vi "Auto.vi"() -> ()   [LabVIEW 2020]
uses:
  Global_Variable/A180648.vi
  Global_Variable/Global.vi
  Global_Variable/excursion.vi
  <userlib>/_MGI/1D Array/MGI Running Average/MGI Running Average(DBL).vi
  <userlib>/_MGI/1D Array/MGI Running Average/MGI Running Average(SGL).vi
  <userlib>/_MGI/1D Array/MGI Average/MGI Average (DBL[][]).vi
  Libraries/S7/S7.lvlib
  <vilib>/ptbypt/NI_PtbyPt.lvlib
panel:
  out "可信度检测":cluster{dbl[], dbl[]}[](graph)
  out "传感器特性":cluster{dbl[], dbl[]}[](graph)
  in  "error in (no error)":errorcluster caption="错误输入（无错误）"
  out "初始角度":dbl
  out "T1-T2_135°":dbl
  out "T1-T2_225°":dbl
  out "T1-T2_315°":dbl
  out "T1-T2_360°":dbl
  out "T1-T2_270°":dbl
  out "T1-T2_180°":dbl
  out "T1-T2_45°":dbl
  out "T1-T2_90°":dbl
  out "初始化 3":bool[](array[boolean])
  out "动优化态前":cluster{dbl[], dbl[]}[](graph)
  in  "initialize 2":bool caption="初始化"
  in  "initialize":bool caption="初始化"
  out "vRES_cCW":cluster{dbl[], dbl[]}
  out "VRES_cW":cluster{dbl[], dbl[]}
  out "初始化 2":bool[](array[boolean])
  in  "选项卡控件":enum32{"工位一程序复检", "工位一动态复检"}(tab)
  in  "请启动":bool
  out "Vres_45°":dbl format="%#.6f"
  out "Vres_135°":dbl format="%#.6f"
  out "Vres_225°":dbl format="%#.6f"
  out "Vres_315°":dbl format="%#.6f"
  out "Vres_360°":dbl format="%#.6f"
  out "Vres_270°":dbl format="%#.6f"
  out "Vres_180°":dbl format="%#.6f"
  out "Vres_90°":dbl format="%#.6f"
  out "S_CCw":dbl[](array[numeric]) caption="数据" format="%0.6f"
  out "P_CCw":dbl[](array[numeric]) caption="数据" format="%0.6f"
  out "S_CW":dbl[](array[numeric]) caption="数据" format="%0.6f"
  out "P_CW":dbl[](array[numeric]) caption="数据" format="%0.6f"
  out "T1_CCw":dbl[](array[numeric]) caption="数据" format="%0.2f"
  out "T2_CCw":dbl[](array[numeric]) caption="数据" format="%0.2f"
  out "T2_CW":dbl[](array[numeric]) caption="数据" format="%0.2f"
  out "T1_CW":dbl[](array[numeric]) caption="数据" format="%0.2f"
  out "初始化":bool[](array[boolean])
  out "SENSOR":T1
  in  "判定结果":bool[][](array[boolean])=[[TRUE]]
  in  "STEP":string
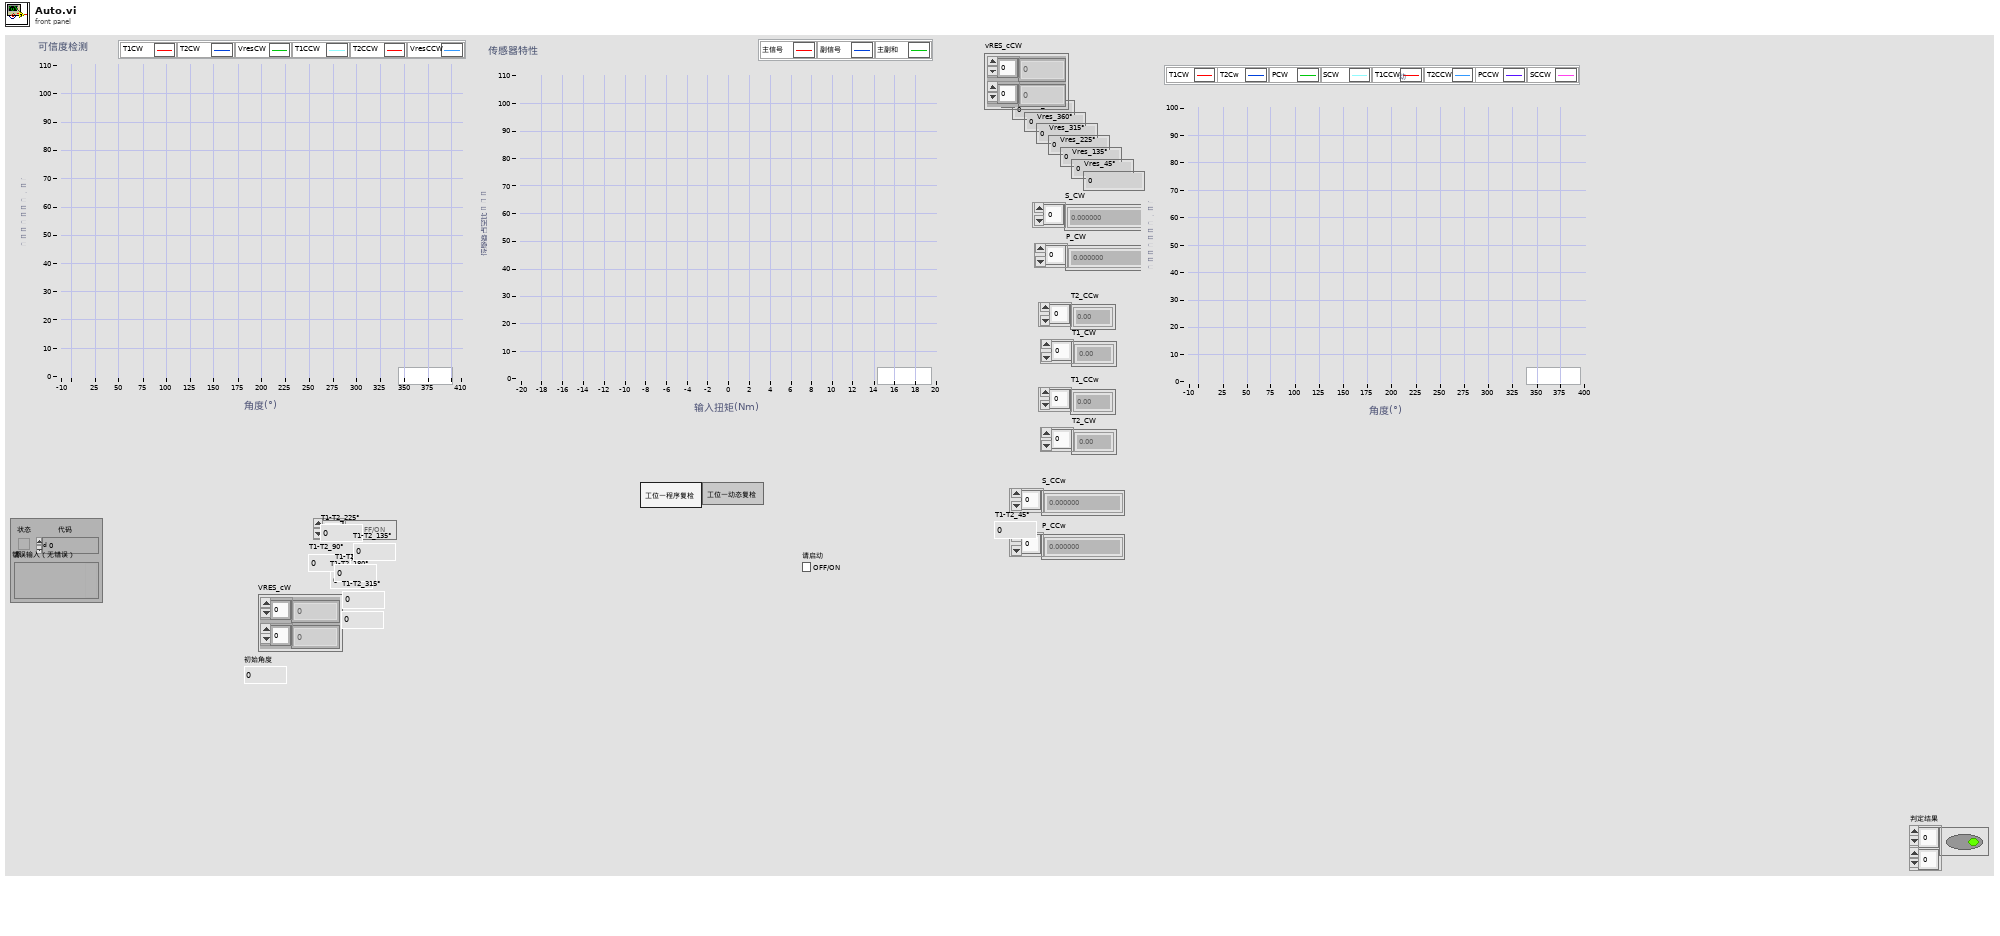
[diagram p1: front panel]
types:
  T1 = cluster{"hSENSOR":i32, "hASIC_T1":i32, "hASIC_T2":i32, "hASIC_P":i32, "hASIC_S":i32}
  T2 = typedef "检测CTR.xctl/检测CTR数据.ctl" = enum16{"Idle", "Runing", "Pass", "Faild", "Skip"}
  T3 = enum32{"Invalid", "Standard", "Closed", "Hidden", "Minimized", "Maximized"}
  T4 = enum16{"Idle", "Runing", "Pass", "Faild", "Skip"}
  T5 = enum16{"open", "replace", "create", "open or create", "replace or create", "replace or create with confirmation"}
  T6 = cluster{"工位一驱动伺服位移":sgl, "工位二驱动伺服位移":sgl, "工位一移载伺服位移":sgl, "工位二移载伺服位移":sgl, "工位一编码器位移":sgl, "工位二编码器位移":sgl, "工位一扭矩":sgl, "工位二扭矩":sgl}
  T7 = typedef "System_conf.ctl" = cluster{"右上升":dbl, "右下降":dbl, "左上升":dbl, "左下降":dbl, "左逆向":dbl, "左正向":dbl}
  T8 = cluster{"主副信号和MAX":cluster{"单位":string, "下限":dbl, "上限":dbl}, "主副信号和MIN":cluster{"单位":string, "下限":dbl, "上限":dbl}, "主信号线性误差":cluster{"单位":string, "下限":dbl, "上限":dbl}, "副信号线性误差":cluster{"单位":string, "下限":dbl, "上限":dbl}, "主信号MAX":cluster{"单位":string, "下限":dbl, "上限":dbl}, "主信号MIN":cluster{"单位":string, "下限":dbl, "上限":dbl}, "副信号MAX":cluster{"单位":string, "下限":dbl, "上限":dbl}, "副信号MIN":cluster{"单位":string, "下限":dbl, "上限":dbl}, "中心偏移量":cluster{"单位":string, "下限":dbl, "上限":dbl}, "定点设置":cluster{"单位":string, "下限":dbl, "上限":dbl}, "定点左侧主信号":cluster{"单位":string, "下限":dbl, "上限":dbl}, "定点左侧副信号":cluster{"单位":string, "下限":dbl, "上限":dbl}, "定点右侧主信号":cluster{"单位":string, "下限":dbl, "上限":dbl}, "定点右侧副信号":cluster{"单位":string, "下限":dbl, "上限":dbl}, "监测点1左滞后":cluster{"单位":string, "下限":dbl, "上限":dbl}, "监测点1右滞后":cluster{"单位":string, "下限":dbl, "上限":dbl}, "监测点2左滞后":cluster{"单位":string, "下限":dbl, "上限":dbl}, "监测点2右滞后":cluster{"单位":string, "下限":dbl, "上限":dbl}, "监测点3左滞后":cluster{"单位":string, "下限":dbl, "上限":dbl}, "监测点3右滞后":cluster{"单位":string, "下限":dbl, "上限":dbl}}
  T9 = cluster{"复检速度":dbl, "换向扭矩":dbl, "判定范围下限":dbl, "判定范围上限":dbl, "滞后监测点1":dbl, "滞后监测点2":dbl, "滞后监测点3":dbl}
  T10 = cluster{"可信度检测":cluster{dbl[], dbl[]}[], "动优化态前":cluster{dbl[], dbl[]}[], "传感器特性":cluster{dbl[], dbl[]}[]}
  T11 = typedef "lveventtype.ctl" = enum32{"Null", "Timeout", "Annotation Menu Selection", "Annotation Menu Selection?", "App Instance Close", "App Instance Close?", "Autoscale Range Change", "Bookmark Info Change", "Cell Edit", "Cell Edit?", "Cursor Grab", "Cursor Grab?", "Cursor Menu Selection", "Cursor Menu Selection?", "Cursor Move", "Cursor Release", "Data Change", "Direction Change", "Display State Change", "Drag Ended", "Drag Enter", "Drag Leave", "Drag Over", "Drag Source Update", "Drag Starting", "Drag Starting?", "Drop", "Exec State Change", "Key Down", "Key Down?", "Key Repeat", "Key Repeat?", "Key Up", "Listbox Double Click", "Menu Activation?", "Menu Selection (App)", "Menu Selection? (App)", "Menu Selection (User)", "Mouse Down", "Mouse Down?", "Mouse Enter", "Mouse Leave", "Mouse Move", "Mouse Up", "Mouse Wheel", "NI Security User Change (App)", "Pane Size", "Panel Close", "Panel Close?", "Panel Resize", "Plot Attribute Change", "Scale Range Change", "Shortcut Menu Activation?", "Shortcut Menu Selection (App)", "Shortcut Menu Selection? (App)", "Shortcut Menu Selection (User)", "Tree Double Click", "Tree Drag", "Tree Drag?", "Tree Drop", "Tree Drop?", "Tree Item Close", "Tree Item Close?", "Tree Item Open", "Tree Item Open?", "User Event", "Value Change"}
  T12 = typedef "LVPoint32TypeDef.ctl" = cluster{"Horizontal":i32, "Vertical":i32}
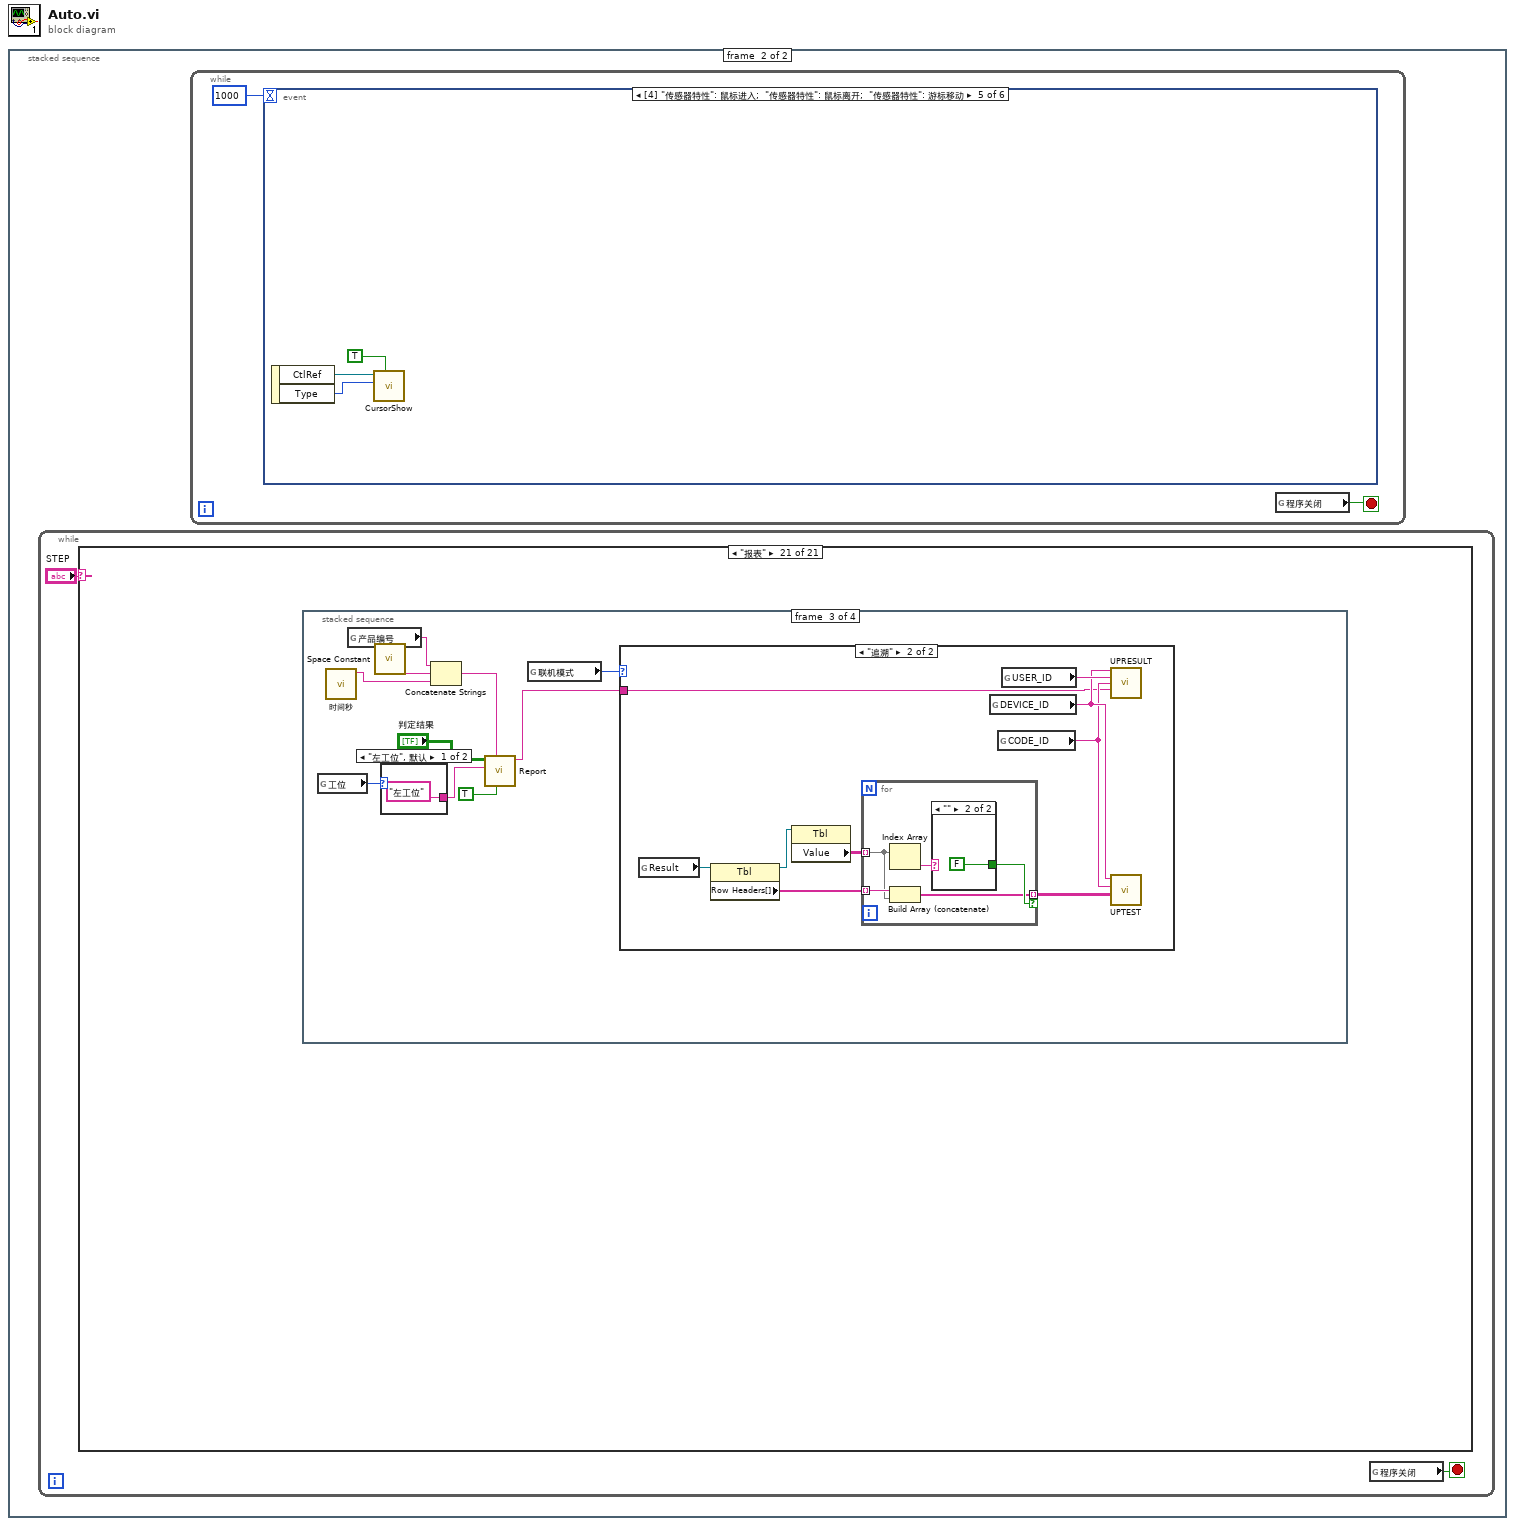
[diagram p0: block diagram]
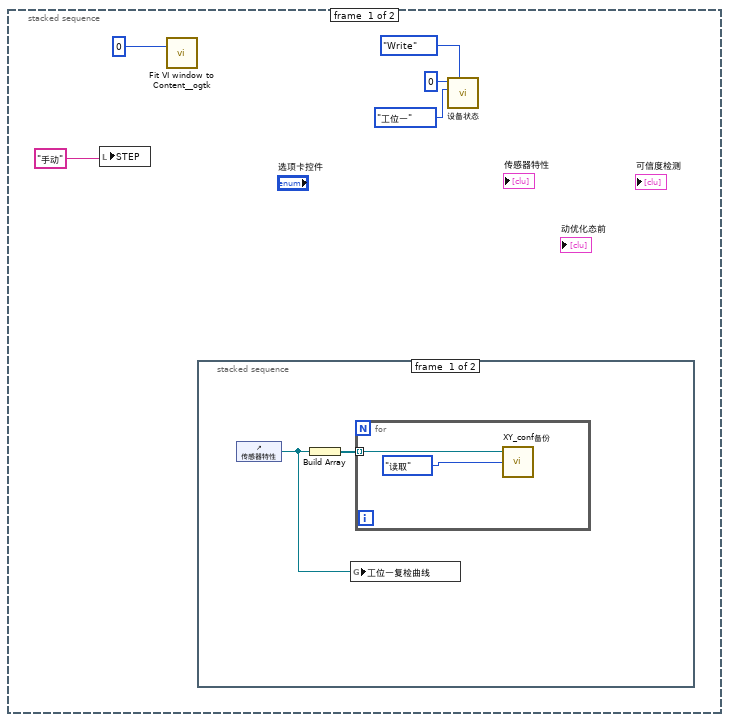
[diagram p2: hidden frame]
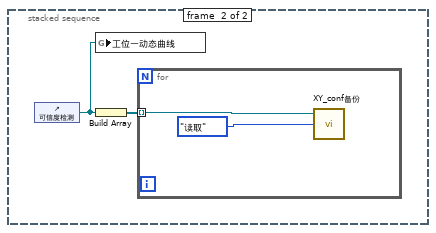
[diagram p3: hidden frame]
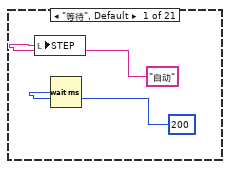
[diagram p4: hidden frame]
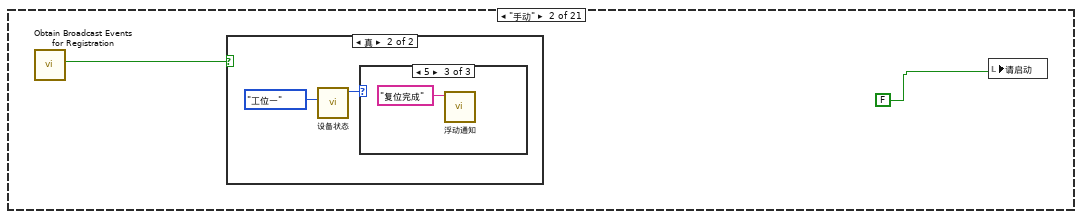
[diagram p5: hidden frame]
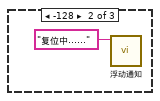
[diagram p8: hidden frame]
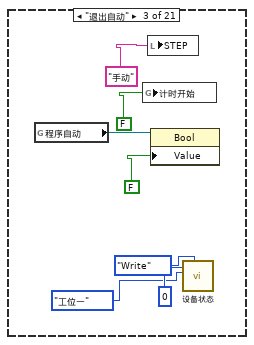
[diagram p9: hidden frame]
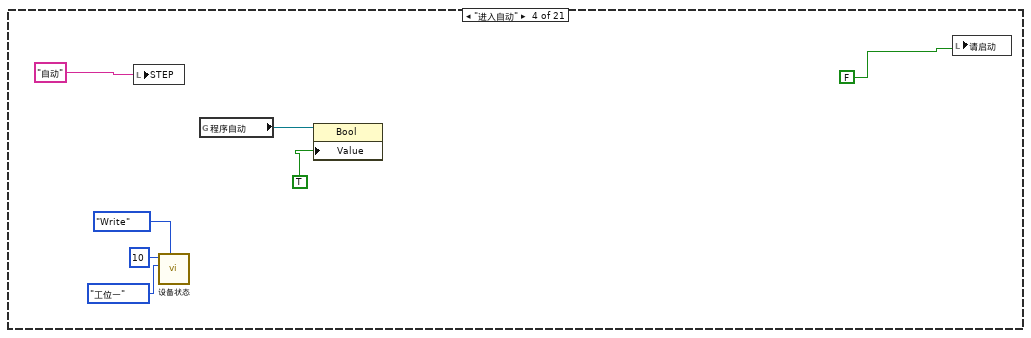
[diagram p10: hidden frame]
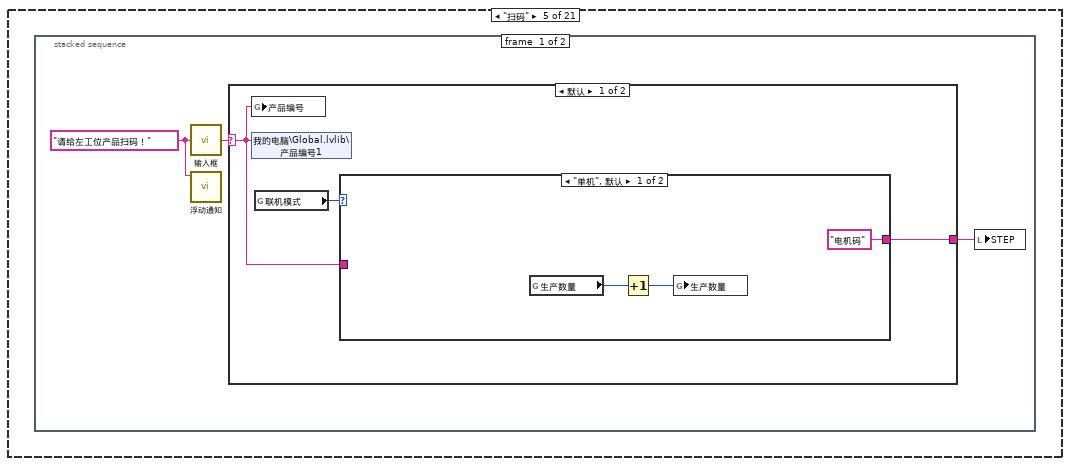
[diagram p11: hidden frame]
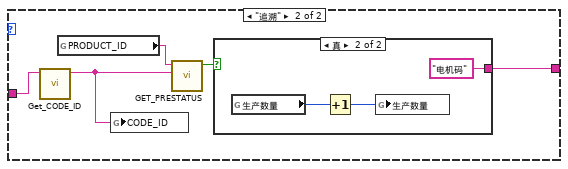
[diagram p12: hidden frame]
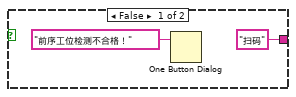
[diagram p13: hidden frame]
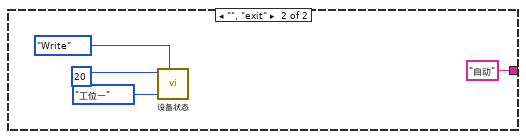
[diagram p14: hidden frame]
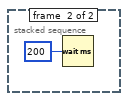
[diagram p15: hidden frame]
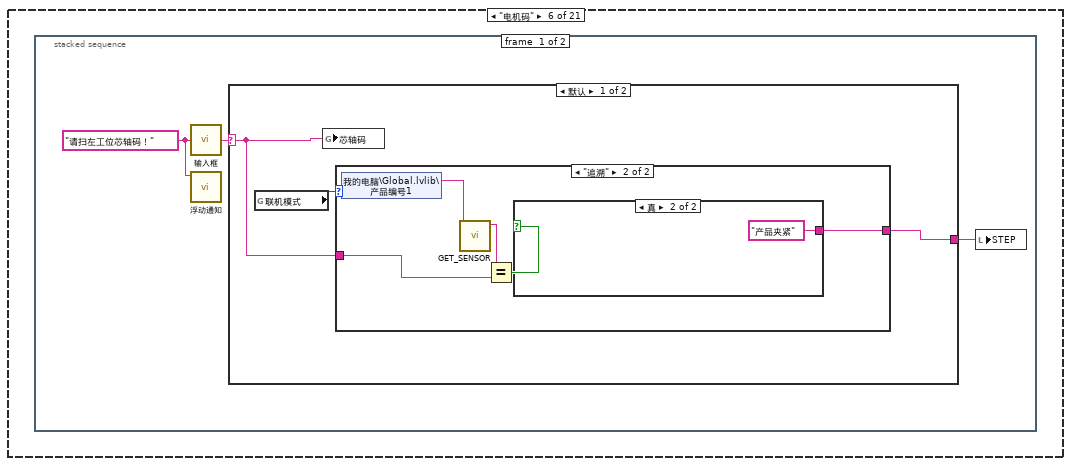
[diagram p16: hidden frame]
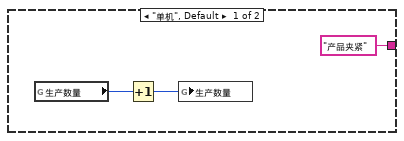
[diagram p17: hidden frame]
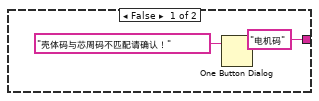
[diagram p18: hidden frame]
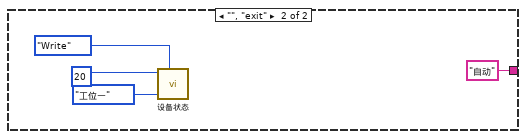
[diagram p19: hidden frame]
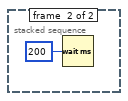
[diagram p20: hidden frame]
diagram:
  n1 = stacked-sequence {
    frame #0 {
      n2 = local write "STEP"("手动" ("STEP")) -> ()
      n3 = call <userlib>:"Fit VI window to Content__ogtk.vi"("border spacing (2 px)"=0) -> ()  [unwired: 5 in, 2 out]
      n4 = stacked-sequence {
        frame #0 {
          n5 = control-ref of="传感器特性"() -> (w6:refnum<vi>)
          n6 = Build Array(w6) -> (w7:refnum<vi>[])
          n7 = global write "A180648.vi" "工位一复检曲线"(w6) -> ()
          n8 = for {
            tunnel: w7 -> [w8] mode=indexing
            n9 = call "XY_conf备份.vi"("方式"=enum16{"写入", "读取"}."读取", "XY图引用"=w8) -> ()  [unwired: 3 in, 1 out]
          }
        }
        frame #1 {
          n10 = control-ref of="可信度检测"() -> (w11:refnum<vi>)
          n11 = global write "A180648.vi" "工位一动态曲线"(w11) -> ()
          n12 = Build Array(w11) -> (w10:refnum<vi>[])
          n13 = for {
            tunnel: w10 -> [w12] mode=indexing
            n14 = call "XY_conf备份.vi"("方式"=enum16{"写入", "读取"}."读取", "XY图引用"=w12) -> ()  [unwired: 3 in, 1 out]
          }
        }
      }
      n15 = call "设备状态.vi"("枚举"=enum16{"Read", "Write"}."Write", "工位"=enum16{"工位一", "工位二"}."工位一", "Status_Write"=i16 0) -> ()  [unwired: 8 in, 1 out]
    }
    frame #1 {
      n16 = while {
        stop <- w15 stop-if-true
        n17 = case shown="\"报表\"" "STEP" {
          frame "等待", Default {
            n18 = local write "STEP"("自动" ("STEP")) -> ()
            n19 = Wait (ms)(milliseconds to wait=u32 200 ("等待时间（毫秒）")) -> ()  [unwired: 1 out]
          }
          frame "手动" {
            n20 = call "Obtain Broadcast Events for Registration.vi"() -> ("Already running?"=w19:bool)  [unwired: 9 in, 2 out]
            n21 = case shown="真" w19 {
              frame False {
              }
              frame True {
                n22 = call "设备状态.vi"("工位"=enum16{"工位一", "工位二"}."工位一") -> ("Status_Read"=w21:i16)  [unwired: 10 in]
                n23 = case shown="5" w21 {
                  frame 0, Default {
                  }
                  frame -128 {
                    n24 = call "浮动通知.vi"("通知内容"="复位中……" ("Status")) -> ()  [unwired: 11 in]
                  }
                  frame 5 {
                    n25 = call "浮动通知.vi"("通知内容"="复位完成" ("Status")) -> ()  [unwired: 11 in]
                  }
                }
              }
            }
            n26 = local write "请启动"(FALSE ("请启动")) -> ()
          }
          frame "退出自动" {
            n27 = global read "Global.vi" "程序自动"() -> (w26:refnum<vi>)
            n28 = global write "Global.vi" "计时开始"(FALSE ("计时开始")) -> ()
            n29 = local write "STEP"("手动" ("STEP")) -> ()
            n30 = property class="Bool"(reference=w26, "Value"=FALSE) -> ()  [unwired: 1 in, 2 out]
            n31 = call "设备状态.vi"("枚举"=enum16{"Read", "Write"}."Write", "工位"=enum16{"工位一", "工位二"}."工位一", "Status_Write"=i16 0) -> ()  [unwired: 8 in, 1 out]
          }
          frame "进入自动" {
            n32 = local write "STEP"("自动" ("STEP")) -> ()
            n33 = call "设备状态.vi"("枚举"=enum16{"Read", "Write"}."Write", "工位"=enum16{"工位一", "工位二"}."工位一", "Status_Write"=i16 10) -> ()  [unwired: 8 in, 1 out]
            n34 = global read "Global.vi" "程序自动"() -> (w36:refnum<vi>)
            n35 = property class="Bool"(reference=w36, "Value"=TRUE) -> ()  [unwired: 1 in, 2 out]
            n36 = local write "请启动"(FALSE ("请启动")) -> ()
          }
          frame "扫码" {
            n37 = stacked-sequence {
              frame #0 {
                w39 = "请给左工位产品扫码！" ("提示信息")
                n38 = call "输入框.vi"("提示信息"=w39) -> ("条形码输出"=w40:string)
                n39 = call "浮动通知.vi"("通知内容"=w39) -> ()  [unwired: 11 in]
                n40 = case shown="默认" w40 {
                  selector: w40 -> [w41 _]
                  tunnel: [w43 "自动" ("State(s) in Front (\"\")")] -> w38
                  frame Default {
                    n41 = global write "Global.vi" "产品编号"(w41) -> ()
                    n42 = shared-variable "我的电脑\\Global.lvlib\\产品编号1"(w41) -> ()  [unwired: 1 in, 1 out]
                    n43 = global read "Global.vi" "联机模式"() -> (w42:enum16{"单机", "追溯"})
                    n44 = case shown="\"单机\", 默认" w42 {
                      tunnel: ["电机码" ("State(s) in Front (\"\")") w51] -> w43
                      tunnel: w41 -> [_ w48]
                      frame "单机", Default {
                        n45 = global read "Global.vi" "生产数量"() -> (w44:i32)
                        n46 = Increment(x=w44) -> (x+1=w45:i32)
                        n47 = global write "Global.vi" "生产数量"(w45) -> ()
                      }
                      frame "追溯" {
                        n48 = call "Get_CODE_ID.vi"("CODE_MAIN"=w48) -> ("CODE_ID"=w47:string)  [unwired: 10 in]
                        n49 = global read "追溯Global.vi" "PRODUCT_ID"() -> (w50:string)
                        n50 = global write "追溯Global.vi" "CODE_ID"(w47) -> ()
                        n51 = call "GET_PRESTATUS.vi"("CODE_ID"=w47, "PRODUCT_ID"=w50) -> ("OK?"=w49:bool)  [unwired: 9 in]
                        n52 = case shown="真" w49 {
                          tunnel: ["扫码" ("State(s) in Front (\"\")") "电机码" ("State(s) in Front (\"\")")] -> w51
                          frame False {
                            n53 = One Button Dialog(message="前序工位检测不合格！" ("消息")) -> ()  [unwired: 1 in, 1 out]
                          }
                          frame True {
                            n54 = global read "Global.vi" "生产数量"() -> (w54:i32)
                            n55 = Increment(x=w54) -> (x+1=w55:i32)
                            n56 = global write "Global.vi" "生产数量"(w55) -> ()
                          }
                        }
                      }
                    }
                  }
                  frame "", "exit" {
                    n57 = call "设备状态.vi"("枚举"=enum16{"Read", "Write"}."Write", "工位"=enum16{"工位一", "工位二"}."工位一", "Status_Write"=i16 20) -> ()  [unwired: 8 in, 1 out]
                  }
                }
                n58 = local write "STEP"(w38) -> ()
              }
              frame #1 {
                n59 = Wait (ms)(milliseconds to wait=u32 200 ("等待时间（毫秒）")) -> ()  [unwired: 1 out]
              }
            }
          }
          frame "电机码" {
            n60 = stacked-sequence {
              frame #0 {
                w63 = "请扫左工位芯轴码！" ("提示信息")
                n61 = call "输入框.vi"("提示信息"=w63) -> ("条形码输出"=w64:string)
                n62 = call "浮动通知.vi"("通知内容"=w63) -> ()  [unwired: 11 in]
                n63 = case shown="默认" w64 {
                  selector: w64 -> [w65 _]
                  tunnel: [w67 "自动" ("State(s) in Front (\"\")")] -> w62
                  frame Default {
                    n64 = global read "Global.vi" "联机模式"() -> (w66:enum16{"单机", "追溯"})
                    n65 = global write "Global.vi" "芯轴码"(w65) -> ()
                    n66 = case shown="\"追溯\"" w66 {
                      tunnel: ["产品夹紧" ("State(s) in Front (\"\")") w75] -> w67
                      tunnel: w65 -> [_ w72]
                      frame "单机", Default {
                        n67 = global read "Global.vi" "生产数量"() -> (w68:i32)
                        n68 = Increment(x=w68) -> (x+1=w69:i32)
                        n69 = global write "Global.vi" "生产数量"(w69) -> ()
                      }
                      frame "追溯" {
                        n70 = shared-variable "我的电脑\\Global.lvlib\\产品编号1"() -> (w74:string)  [unwired: 1 in, 1 out]
                        n71 = call "GET_SENSOR.vi"("CODE_MAIN"=w74) -> ("CODE_MOTOR"=w73:string)  [unwired: 10 in]
                        n72 = Equal?(x=w73, y=w72) -> (x = y?=w71:bool)
                        n73 = case shown="真" w71 {
                          tunnel: ["电机码" ("State(s) in Front (\"\")") "产品夹紧" ("State(s) in Front (\"\")")] -> w75
                          frame False {
                            n74 = One Button Dialog(message="壳体码与芯周码不匹配请确认！" ("消息")) -> ()  [unwired: 1 in, 1 out]
                          }
                          frame True {
                          }
                        }
                      }
                    }
                  }
                  frame "", "exit" {
                    n75 = call "设备状态.vi"("枚举"=enum16{"Read", "Write"}."Write", "工位"=enum16{"工位一", "工位二"}."工位一", "Status_Write"=i16 20) -> ()  [unwired: 8 in, 1 out]
                  }
                }
                n76 = local write "STEP"(w62) -> ()
              }
              frame #1 {
                n77 = Wait (ms)(milliseconds to wait=u32 200 ("等待时间（毫秒）")) -> ()  [unwired: 1 out]
              }
            }
          }
          frame "传感器码" {
            n78 = stacked-sequence {
              frame #0 {
                w85 = "请给左工位产品扫码！" ("提示信息")
                n79 = call "输入框.vi"("提示信息"=w85) -> ("条形码输出"=w86:string)
                n80 = call "浮动通知.vi"("通知内容"=w85) -> ()  [unwired: 11 in]
                n81 = case shown="\"\", \"exit\"" w86 {
                  selector: w86 -> [w87 _]
                  tunnel: [w89 "自动" ("State(s) in Front (\"\")")] -> w84
                  frame Default {
                    n82 = global write "Global.vi" "产品编号"(w87) -> ()
                    n83 = shared-variable "我的电脑\\Global.lvlib\\产品编号1"(w87) -> ()  [unwired: 1 in, 1 out]
                    n84 = global read "Global.vi" "联机模式"() -> (w88:enum16{"单机", "追溯"})
                    n85 = case shown="\"追溯\"" w88 {
                      tunnel: ["产品夹紧" ("State(s) in Front (\"\")") w97] -> w89
                      tunnel: w87 -> [_ w94]
                      frame "单机", Default {
                        n86 = global read "Global.vi" "生产数量"() -> (w90:i32)
                        n87 = Increment(x=w90) -> (x+1=w91:i32)
                        n88 = global write "Global.vi" "生产数量"(w91) -> ()
                      }
                      frame "追溯" {
                        n89 = call "Get_CODE_ID_Sensor.vi"("CODE_SENSOR"=w94) -> ("CODE_ID"=w93:string)  [unwired: 10 in]
                        n90 = global read "追溯Global.vi" "PRODUCT_ID"() -> (w96:string)
                        n91 = global write "追溯Global.vi" "CODE_ID"(w93) -> ()
                        n92 = call "GET_PRESTATUS.vi"("CODE_ID"=w93, "PRODUCT_ID"=w96) -> ("OK?"=w95:bool)  [unwired: 9 in]
                        n93 = case shown="假" w95 {
                          tunnel: ["传感器码" ("State(s) in Front (\"\")") "产品夹紧" ("State(s) in Front (\"\")")] -> w97
                          frame False {
                            n94 = One Button Dialog(message="前序工位检测不合格！" ("消息")) -> ()  [unwired: 1 in, 1 out]
                          }
                          frame True {
                            n95 = global read "Global.vi" "生产数量"() -> (w100:i32)
                            n96 = Increment(x=w100) -> (x+1=w101:i32)
                            n97 = global write "Global.vi" "生产数量"(w101) -> ()
                          }
                        }
                      }
                    }
                  }
                  frame "", "exit" {
                    n98 = call "设备状态.vi"("枚举"=enum16{"Read", "Write"}."Write", "工位"=enum16{"工位一", "工位二"}."工位一", "Status_Write"=i16 20) -> ()  [unwired: 8 in, 1 out]
                  }
                }
                n99 = local write "STEP"(w84) -> ()
              }
              frame #1 {
                n100 = Wait (ms)(milliseconds to wait=u32 200 ("等待时间（毫秒）")) -> ()  [unwired: 1 out]
              }
            }
          }
          frame "产品夹紧" {
            n101 = stacked-sequence {
              frame #0 {
                n102 = case shown="真" "请启动" {
                  frame False {
                    n103 = call "浮动通知.vi"("通知内容"="请启动工左位" ("Status")) -> ()  [unwired: 11 in]
                    n104 = call "设备状态.vi"("枚举"=enum16{"Read", "Write"}."Write", "工位"=enum16{"工位一", "工位二"}."工位一", "Status_Write"=i16 99) -> ()  [unwired: 8 in, 1 out]
                    n105 = local write "请启动"(TRUE ("请启动")) -> ()
                  }
                  frame True {
                  }
                }
              }
              frame #1 {
                n106 = call "设备状态.vi"("工位"=enum16{"工位一", "工位二"}."工位一") -> ("Status_Read"=w114:i16)  [unwired: 10 in]
                n107 = case shown="0, 默认" w114 {
                  frame 0, Default {
                  }
                  frame 100 {
                    n108 = local write "STEP"("初始化") -> ()
                    n109 = local write "请启动"(FALSE ("请启动")) -> ()
                  }
                }
              }
            }
          }
          frame "套输入轴" {
            n110 = global read "Global.vi" "可信度检测引用句柄"() -> (w127:refnum<vi>)
            n111 = global read "Global.vi" "传感器特性用句柄"() -> (w124:refnum<vi>)
            n112 = property class="检测CTR"(reference=w124) -> ("Value"=w125:variant)  [unwired: 1 in, 2 out]
            n113 = property class="检测CTR"(reference=w127) -> ("Value"=w126:variant)  [unwired: 1 in, 2 out]
            n114 = Variant To Data(type=检测CTR数据."Idle" ("Data"), Variant=w125) -> (data=w123:T2)  [unwired: 1 in, 1 out]
            n115 = Variant To Data(type=检测CTR数据."Idle" ("Data"), Variant=w126) -> (data=w128:T2)  [unwired: 1 in, 1 out]
            n116 = Equal?(x=w123, y=检测CTR数据."Skip" ("Data")) -> (x = y?=w129:bool)
            n117 = Equal?(x=w128, y=检测CTR数据."Skip" ("Data")) -> (x = y?=w130:bool)
            n118 = And(x=w129, y=w130) -> (x .and. y?=w118:bool)
            n119 = case shown="假" w118 {
              frame False {
                n120 = stacked-sequence {
                  frame #0 {
                    n121 = call "浮动通知.vi"("通知内容"="左工位产品套输入轴" ("Status")) -> ()  [unwired: 11 in]
                    n122 = call "设备状态.vi"("枚举"=enum16{"Read", "Write"}."Write", "工位"=enum16{"工位一", "工位二"}."工位一", "Status_Write"=i16 112) -> ()  [unwired: 8 in, 1 out]
                    n123 = vi-ref "T1T2占空比.vi"() -> (w134:refnum<vi>)
                    n124 = call "CallVI.vi"("VI引用"=w134, "状态"=T3."Hidden") -> ()  [unwired: 12 in, 2 out]
                    n125 = vi-ref "PS采集优化.vi"() -> (w131:refnum<vi>)
                    n126 = call "CallVI.vi"("VI引用"=w131, "状态"=T3."Hidden") -> ()  [unwired: 12 in, 2 out]
                  }
                  frame #1 {
                    n127 = while {
                      stop <- w139 stop-if-true
                      n128 = call "设备状态.vi"("工位"=enum16{"工位一", "工位二"}."工位一") -> ("Status_Read"=w140:i16)  [unwired: 10 in]
                      n129 = case shown="113" w140 {
                        tunnel: [w142 TRUE] -> w139
                        frame 0, Default {
                          n130 = call "套输入轴时间"() -> ("Time has Elapsed"=w143:bool)  [unwired: 12 in, 7 out]
                          n131 = case shown="真" w143 {
                            tunnel: [FALSE TRUE] -> w142
                            frame False {
                            }
                            frame True {
                              n132 = call "浮动通知.vi"("通知内容"="工位一产品套输入轴超时" ("Status")) -> ()  [unwired: 11 in]
                            }
                          }
                        }
                        frame 113 {
                          n133 = local write "STEP"("动态优化") -> ()
                        }
                      }
                    }
                  }
                }
              }
              frame True {
                n134 = local write "STEP"("程序固化" ("STEP")) -> ()
              }
            }
          }
          frame "套输出轴" {
            n135 = global read "Global.vi" "传感器特性用句柄"() -> (w154:refnum<vi>)
            n136 = property class="检测CTR"(reference=w154) -> ("Value"=w153:variant)  [unwired: 1 in, 2 out]
            n137 = Variant To Data(type=检测CTR数据."Idle" ("Data"), Variant=w153) -> (data=w155:T2)  [unwired: 1 in, 1 out]
            n138 = Equal?(x=w155, y=检测CTR数据."Skip" ("Data")) -> (x = y?=w150:bool)
            n139 = case shown="假" w150 {
              frame False {
                n140 = stacked-sequence {
                  frame #0 {
                    n141 = call "设备状态.vi"("枚举"=enum16{"Read", "Write"}."Write", "工位"=enum16{"工位一", "工位二"}."工位一", "Status_Write"=i16 108) -> ()  [unwired: 8 in, 1 out]
                    n142 = call "浮动通知.vi"("通知内容"="左工位产品套输出轴" ("Status")) -> ()  [unwired: 11 in]
                  }
                  frame #1 {
                    n143 = while {
                      stop <- w160 stop-if-true
                      n144 = call "设备状态.vi"("工位"=enum16{"工位一", "工位二"}."工位一") -> ("Status_Read"=w161:i16)  [unwired: 10 in]
                      n145 = case shown="109" w161 {
                        tunnel: [w163 TRUE] -> w160
                        frame 0, Default {
                          n146 = call "套输出轴时间"() -> ("Time has Elapsed"=w164:bool)  [unwired: 12 in, 7 out]
                          n147 = case shown="真" w164 {
                            tunnel: [FALSE TRUE] -> w163
                            frame False {
                            }
                            frame True {
                              n148 = call "浮动通知.vi"("通知内容"="左工位产品套输出轴超时" ("Status")) -> ()  [unwired: 11 in]
                            }
                          }
                        }
                        frame 109 {
                          n149 = global read "Global.vi" "产品型号"() -> (w168:string)
                          n150 = call "传感器数据.vi"() -> ("传感器读数"=w170:T6)  [unwired: 11 in]
                          n151 = Unbundle By Name(w170) -> ("工位一驱动伺服位移"=→"初始角度":sgl)
                          n152 = case shown="\"真\", 默认" w168 {
                            tunnel: ["等待" "程序复检"] -> w172
                            frame "R567X" {
                              n153 = call "设备状态.vi"("枚举"=enum16{"Read", "Write"}."Write", "工位"=enum16{"工位一", "工位二"}."工位一", "Status_Write"=i16 400) -> ()  [unwired: 8 in, 1 out]
                            }
                            frame "真", Default {
                            }
                          }
                          n154 = local write "STEP"(w172) -> ()
                        }
                      }
                    }
                  }
                }
              }
              frame True {
                n155 = local read "判定结果"() -> (w180:bool[][])
                n156 = global read "Global.vi" "产品型号"() -> (w178:string)
                n157 = Build Array (concatenate)(w180, bool[][] [[FALSE, TRUE]] ("判定结果")) -> (w181:bool[][])
                n158 = local write "判定结果"(w181) -> ()
                n159 = case shown="默认" w178 {
                  tunnel: ["程序固化" ("STEP") "等待"] -> w182
                  frame Default {
                  }
                  frame "R567X" {
                    n160 = call "设备状态.vi"("枚举"=enum16{"Read", "Write"}."Write", "工位"=enum16{"工位一", "工位二"}."工位一", "Status_Write"=i16 400) -> ()  [unwired: 8 in, 1 out]
                  }
                }
                n161 = local write "STEP"(w182) -> ()
              }
            }
          }
          frame "初始化" {
            n162 = stacked-sequence {
              frame #0 {
                w193 = cluster{dbl[], dbl[]} {[], []} ("vRES_cCW")
                n163 = global read "Global.vi" "产品型号"() -> (w188:string)
                n164 = global write "Global.vi" "IO_Stop"(TRUE ("IO_Stop")) -> ()
                n165 = global write "Global.vi" "计时开始"(TRUE ("计时开始")) -> ()
                n166 = global write "Global.vi" "工位占空比采集"(FALSE ("工位二占空比采集")) -> ()
                n167 = call "标定数据保存.vi"("Section"=w188, "枚举"=enum16{"读取", "保存"}."读取") -> ()  [unwired: 10 in]
                n168 = global write "Global.vi" "P/S采集"(FALSE ("工位二占空比采集")) -> ()
                n169 = local write "判定结果"(bool[][] [] ("判定结果")) -> ()
                n170 = call "System_Conf_RW.vi"("Mode"=enum16{"Read", "Write"}."Read", "Section"=w188) -> ("excursion_out"=w191:T7)  [unwired: 8 in, 1 out]
                n171 = global write "excursion.vi" "excursion"(w191) -> ()
                n172 = global write "Global.vi" "动态优化完成"(FALSE ("动态优化完成")) -> ()
                n173 = local write "vRES_cCW"(w193) -> ()
                n174 = local write "VRES_cW"(w193) -> ()
              }
              frame #1 {
                w204 = dbl[] [] ("S_CCw")
                w205 = dbl[] [] ("T1_cw")
                n175 = local write "T1_CW"(w205) -> ()
                n176 = local write "T2_CW"(w205) -> ()
                n177 = local write "P_CW"(w205) -> ()
                n178 = local write "P_CCw"(w205) -> ()
                n179 = for {
                  N: 12 -> [_]
                  tunnel: [cluster{dbl[], dbl[]} {[], []}] -> w203 mode=indexing
                }
                n180 = local write "传感器特性"(w203) -> ()
                n181 = local write "S_CCw"(w204) -> ()
                n182 = local write "S_CW"(w204) -> ()
                n183 = local write "T1_CCw"(w204) -> ()
                n184 = local write "T2_CCw"(w204) -> ()
                n185 = for {
                  N: 8 -> [_]
                  tunnel: [cluster{dbl[], dbl[]} {[], []}] -> w201 mode=indexing
                }
                n186 = for {
                  N: 8 -> [_]
                  tunnel: [cluster{dbl[], dbl[]} {[], []}] -> w200 mode=indexing
                }
                n187 = local write "动优化态前"(w200) -> ()
                n188 = local write "可信度检测"(w201) -> ()
              }
              frame #2 {
                n189 = global read "Global.vi" "Result"() -> (w221:refnum<vi>)
                n190 = property class="Tbl"(reference=w221, "Value"=string[][] []) -> (reference out=w222:refnum<vi>, error out=w223:errorcluster)  [unwired: 1 in]
                n191 = property class="Tbl"(reference=w222, error in=w223, "Row Headers[]"=string[] [] ("列首字符串[]")) -> ()  [unwired: 2 out]
                n192 = Initialize Array(TRUE, 12 ("维数大小")) -> (→"初始化":bool[])
                n193 = Initialize Array(TRUE, 8 ("维数大小")) -> (→"初始化 2":bool[])
                n194 = Initialize Array(TRUE, 8 ("维数大小")) -> (→"初始化 3":bool[])
              }
              frame #3 {
                n195 = global read "Global.vi" "静态标定引用句柄"() -> (w229:refnum<vi>)
                n196 = global read "Global.vi" "程序固化引用句柄"() -> (w228:refnum<vi>)
                n197 = global read "Global.vi" "动态优化引用句柄"() -> (w227:refnum<vi>)
                n198 = global read "Global.vi" "可信度检测引用句柄"() -> (w224:refnum<vi>)
                n199 = global read "Global.vi" "传感器特性用句柄"() -> (w225:refnum<vi>)
                n200 = Build Array(w229, w228, w227, w225, w224) -> (w226:refnum<vi>[])
                n201 = for {
                  tunnel: w226 -> [w239] mode=indexing
                  n202 = property class="检测CTR"(reference=w239) -> (reference out=w238:refnum<vi>, "Value"=w237:variant)  [unwired: 1 in, 1 out]
                  n203 = Variant To Data(type=检测CTR数据."Idle" ("Data"), Variant=w237) -> (data=w235:T2)  [unwired: 1 in, 1 out]
                  n204 = Equal?(x=w235, y=检测CTR数据."Skip" ("Data")) -> (x = y?=w233:bool)
                  n205 = Select(t=检测CTR数据."Skip" ("Data"), s=w233, f=检测CTR数据."Idle" ("Data")) -> (s? t:f=w230:T2)
                  n206 = property class="检测CTR"(reference=w238, "Value"=w230) -> ()  [unwired: 1 in, 2 out]
                }
              }
              frame #4 {
                n207 = local write "STEP"("静态标定" ("STEP")) -> ()
              }
            }
          }
          frame "静态标定" {
            n208 = global read "Global.vi" "静态标定引用句柄"() -> (w245:refnum<vi>)
            n209 = property class="检测CTR"(reference=w245) -> ("Value"=w244:variant)  [unwired: 1 in, 2 out]
            n210 = Variant To Data(type=检测CTR数据."Idle" ("Data"), Variant=w244) -> (data=w246:T2)  [unwired: 1 in, 1 out]
            n211 = Equal?(x=w246, y=检测CTR数据."Skip" ("Data")) -> (x = y?=w241:bool)
            n212 = case shown="假" w241 {
              frame False {
                n213 = stacked-sequence {
                  tunnel: [_ _ _ w264] -> w247
                  frame #0 {
                    n214 = global read "Global.vi" "静态标定引用句柄"() -> (w249:refnum<vi>)
                    n215 = call "浮动通知.vi"("通知内容"="静态标定" ("Status")) -> ()  [unwired: 11 in]
                    n216 = property class="检测CTR"(reference=w249, "Value"=T4."Runing" ("值")) -> ()  [unwired: 1 in, 2 out]
                  }
                  frame #1 {
                    n217 = call "采集切换.vi"("工位"=enum16{"工位一", "工位二"}."工位一", "采集方式"=enum16{"板卡采集", "PGI采集"}."PGI采集") -> ()  [unwired: 10 in]
                  }
                  frame #2 {
                    n218 = Wait (ms)(milliseconds to wait=u32 200 ("等待时间（毫秒）")) -> ()  [unwired: 1 out]
                  }
                  frame #3 {
                    n219 = call "InitPGI.vi"("DeviceNumber"=1, "error in (no error)"="error in (no error)") -> ("SENSOR"=w256:T1, "error out"=w259:errorcluster)  [unwired: 12 in]
                    "SENSOR" <- w256
                    n220 = call "InitProduct.vi"("SENSOR"=w256, "error in (no error)"=w259) -> ("error out"=w257:errorcluster)  [unwired: 12 in, 1 out]
                    n221 = call "浮动通知.vi"("通知内容"="静态标定中..." ("Status")) -> ()  [unwired: 11 in]
                    n222 = call "StaticCalibration.vi"("SENSOR"=w256, "error in (no error)"=w257) -> ("OK？"=w263:bool, "error out"=w255:errorcluster)  [unwired: 9 in, 3 out]
                    n223 = call "Error Converter (ErrCode or Status).vi"("error in (no error)"=w255) -> ("error out"=w254:errorcluster)  [unwired: 10 in]
                    n224 = Unbundle By Name(w254) -> ("source"=w260:string)
                    n225 = case shown="真" w263 {
                      tunnel: [w271 "套输入轴"] -> w264
                      tunnel: w260 -> [w269 _]
                      frame False {
                        n226 = local read "判定结果"() -> (w266:bool[][])
                        n227 = global read "Global.vi" "静态标定引用句柄"() -> (w278:refnum<vi>)
                        n228 = Build Array (concatenate)(w266, bool[][] [[TRUE, FALSE]] ("判定结果")) -> (w267:bool[][])
                        n229 = local write "判定结果"(w267) -> ()
                        n230 = property class="检测CTR"(reference=w278, "Value"=T4."Faild" ("值")) -> ()  [unwired: 1 in, 2 out]
                        n231 = Concatenate Strings("静态标定失败，可能原因:\n" ("字符串"), w269) -> (w268:string)
                        n232 = Two Button Dialog(message=w268, 1:"否" ("F按钮名称（“取消”）"), 2:"是" ("T按钮名称（“确定”）")) -> (T button?=w274:bool)
                        n233 = Select(t="初始化" ("T按钮名称（“确定”）"), s=w274, f="报表" ("F按钮名称（“取消”）")) -> (s? t:f=w271:string)
                      }
                      frame True {
                        n234 = global read "Global.vi" "静态标定引用句柄"() -> (w283:refnum<vi>)
                        n235 = local read "判定结果"() -> (w279:bool[][])
                        n236 = Build Array (concatenate)(w279, bool[][] [[TRUE, TRUE]] ("判定结果")) -> (w281:bool[][])
                        n237 = local write "判定结果"(w281) -> ()
                        n238 = property class="检测CTR"(reference=w283, "Value"=T4."Pass" ("值")) -> ()  [unwired: 1 in, 2 out]
                      }
                    }
                  }
                }
                n239 = local write "STEP"(w247) -> ()
              }
              frame True {
                n240 = local write "STEP"("套输入轴") -> ()
                n241 = local read "判定结果"() -> (w285:bool[][])
                n242 = Build Array (concatenate)(w285, bool[][] [[FALSE, TRUE]] ("判定结果")) -> (w287:bool[][])
                n243 = local write "判定结果"(w287) -> ()
              }
            }
          }
          frame "动态优化" {
            n244 = global read "Global.vi" "可信度检测引用句柄"() -> (w293:refnum<vi>)
            n245 = property class="检测CTR"(reference=w293) -> ("Value"=w292:variant)  [unwired: 1 in, 2 out]
            n246 = Variant To Data(type=检测CTR数据."Idle" ("Data"), Variant=w292) -> (data=w294:T2)  [unwired: 1 in, 1 out]
            n247 = Equal?(x=w294, y=检测CTR数据."Skip" ("Data")) -> (x = y?=w289:bool)
            n248 = case shown="假" w289 {
              frame False {
                n249 = stacked-sequence {
                  frame #0 {
                    n250 = global read "Global.vi" "可信度检测引用句柄"() -> (w297:refnum<vi>)
                    n251 = call "浮动通知.vi"("通知内容"="可信度检测" ("Status")) -> ()  [unwired: 11 in]
                    n252 = property class="检测CTR"(reference=w297, "Value"=T4."Runing" ("值")) -> ()  [unwired: 1 in, 2 out]
                  }
                  frame #1 {
                    n253 = global read "Global.vi" "跳过优化"() -> (w299:bool)
                    n254 = case shown="真" w299 {
                      selector: w299 -> [_ w306]
                      tunnel: ["自动" w304] -> w298
                      frame False {
                        n255 = call "设备状态.vi"("枚举"=enum16{"Read", "Write"}."Write", "工位"=enum16{"工位一", "工位二"}."工位一", "Status_Write"=i16 505) -> ()  [unwired: 8 in, 1 out]
                      }
                      frame True {
                        n256 = global read "Global.vi" "动态优化复测"() -> (w305:bool)
                        n257 = global write "Global.vi" "动态优化完成"(w306) -> ()
                        n258 = case shown="真" w305 {
                          tunnel: [w307 "自动"] -> w304
                          frame False {
                            n259 = global read "Global.vi" "8点复测"() -> (w308:bool)
                            n260 = case shown="真" w308 {
                              tunnel: ["复测判定" "复测"] -> w307
                              frame False {
                              }
                              frame True {
                              }
                            }
                          }
                          frame True {
                            n261 = call "设备状态.vi"("枚举"=enum16{"Read", "Write"}."Write", "工位"=enum16{"工位一", "工位二"}."工位一", "Status_Write"=i16 505) -> ()  [unwired: 8 in, 1 out]
                          }
                        }
                      }
                    }
                    n262 = local write "STEP"(w298) -> ()
                  }
                }
              }
              frame True {
                n263 = local write "STEP"("套输出轴") -> ()
                n264 = local read "判定结果"() -> (w316:bool[][])
                n265 = Build Array (concatenate)(w316, bool[][] [[FALSE, TRUE]] ("判定结果")) -> (w317:bool[][])
                n266 = local write "判定结果"(w317) -> ()
              }
            }
          }
          frame "复测" {
            n267 = stacked-sequence {
              frame #0 {
                n268 = Wait (ms)(milliseconds to wait=u32 300 ("等待时间（毫秒）")) -> ()  [unwired: 1 out]
              }
              frame #1 {
                n269 = local write "STEP"("自动") -> ()
                n270 = call "浮动通知.vi"("通知内容"="复测" ("Status")) -> ()  [unwired: 11 in]
                n271 = call "设备状态.vi"("枚举"=enum16{"Read", "Write"}."Write", "工位"=enum16{"工位一", "工位二"}."工位一", "Status_Write"=i16 510) -> ()  [unwired: 8 in, 1 out]
              }
            }
          }
          frame "复测判定" {
            w325 = FALSE ("工位占空比采集")
            n272 = local read "Vres_90°"() -> (w345:dbl)
            n273 = local read "Vres_180°"() -> (w344:dbl)
            n274 = local read "Vres_270°"() -> (w343:dbl)
            n275 = local read "Vres_360°"() -> (w342:dbl)
            n276 = local read "Vres_315°"() -> (w337:dbl)
            n277 = local read "Vres_225°"() -> (w336:dbl)
            n278 = local read "Vres_135°"() -> (w335:dbl)
            n279 = local read "Vres_45°"() -> (w341:dbl)
            n280 = local read "T1-T2_90°"() -> (w334:dbl)
            n281 = local read "T1-T2_180°"() -> (w333:dbl)
            n282 = local read "T1-T2_270°"() -> (w332:dbl)
            n283 = local read "T1-T2_360°"() -> (w328:dbl)
            n284 = local read "T1-T2_315°"() -> (w329:dbl)
            n285 = local read "T1-T2_225°"() -> (w330:dbl)
            n286 = local read "T1-T2_135°"() -> (w331:dbl)
            n287 = local read "T1-T2_45°"() -> (w340:dbl)
            n288 = Build Array(w345, w344, w343, w342, w337, w336, w335, w341) -> (w326:dbl[])
            n289 = Build Array(w334, w333, w332, w328, w329, w330, w331, w340) -> (w339:dbl[])
            n290 = Absolute Value(x=w339) -> (abs(x)=w338:dbl[])
            n291 = disable-structure shown="禁用" {
              frame Disabled {
                n292 = Two Button Dialog(message="复测失败\n请选择是否继续？" ("消息"), 1:"否" ("F按钮名称（“取消”）"), 2:"是" ("T按钮名称（“确定”）")) -> ()  [unwired: 1 out]
                n293 = case shown="真" {
                  selector: _ -> [_ _]
                  frame False {
                  }
                  frame True {
                    n294 = local write "STEP"("套输出轴" ("T按钮名称（“确定”）")) -> ()
                  }
                }
              }
              frame Enabled {
              }
            }
            n295 = call "动态优化复测判定.vi"("T1-T2"=w338, "Vres"=w326) -> ("结果1"=w327:bool)  [unwired: 9 in]
            n296 = case shown="真" w327 {
              frame False {
                w353 = enum16{"Read", "Write"}."Write" ("枚举")
                w352 = enum16{"工位一", "工位二"}."工位一" ("工位")
                n297 = global read "Global.vi" "可信度检测引用句柄"() -> (w350:refnum<vi>)
                n298 = local read "判定结果"() -> (w356:bool[][])
                n299 = Build Array (concatenate)(w356, bool[][] [[TRUE, FALSE]] ("判定结果")) -> (w357:bool[][])
                n300 = local write "判定结果"(w357) -> ()
                n301 = property class="检测CTR"(reference=w350, "Value"=T4."Faild" ("值")) -> ()  [unwired: 1 in, 2 out]
                n302 = local write "STEP"("报表" ("F按钮名称（“取消”）")) -> ()
                n303 = call "设备状态.vi"("枚举"=w353, "工位"=w352, "Status_Write"=i16 400) -> ()  [unwired: 8 in, 1 out]
                n304 = call "合格状态.vi"("枚举"=w353, "工位"=w352, "Status_Write"=i16 2) -> ()  [unwired: 8 in, 1 out]
              }
              frame True {
                n305 = global read "Global.vi" "可信度检测引用句柄"() -> (w364:refnum<vi>)
                n306 = local read "判定结果"() -> (w360:bool[][])
                n307 = local write "STEP"("套输出轴") -> ()
                n308 = Build Array (concatenate)(w360, bool[][] [[TRUE, TRUE]] ("判定结果")) -> (w361:bool[][])
                n309 = local write "判定结果"(w361) -> ()
                n310 = property class="检测CTR"(reference=w364, "Value"=T4."Pass" ("值")) -> ()  [unwired: 1 in, 2 out]
              }
            }
            n311 = global write "Global.vi" "工位占空比采集"(w325) -> ()
            n312 = global write "Global.vi" "P/S采集"(w325) -> ()
          }
          frame "程序固化" {
            n313 = global read "Global.vi" "程序固化引用句柄"() -> (w370:refnum<vi>)
            n314 = property class="检测CTR"(reference=w370) -> ("Value"=w369:variant)  [unwired: 1 in, 2 out]
            n315 = Variant To Data(type=检测CTR数据."Idle" ("Data"), Variant=w369) -> (data=w371:T2)  [unwired: 1 in, 1 out]
            n316 = Equal?(x=w371, y=检测CTR数据."Skip" ("Data")) -> (x = y?=w366:bool)
            n317 = case shown="假" w366 {
              frame False {
                n318 = stacked-sequence {
                  frame #0 {
                    n319 = global read "Global.vi" "程序固化引用句柄"() -> (w375:refnum<vi>)
                    n320 = property class="检测CTR"(reference=w375, "Value"=T4."Runing" ("值")) -> ()  [unwired: 1 in, 2 out]
                    n321 = call "设备状态.vi"("枚举"=enum16{"Read", "Write"}."Write", "工位"=enum16{"工位一", "工位二"}."工位一", "Status_Write"=i16 200) -> ()  [unwired: 8 in, 1 out]
                  }
                  frame #1 {
                    n322 = Wait (ms)(milliseconds to wait=u32 500 ("等待时间（毫秒）")) -> ()  [unwired: 1 out]
                  }
                  frame #2 {
                    n323 = local read "SENSOR"() -> (w381:T1)
                    n324 = call "FirmwareProgramming.vi"("SENSOR"=w381) -> ("Message"=w379:string, "Done?"=w380:bool)  [unwired: 8 in, 1 out]
                    n325 = case shown="真" w380 {
                      tunnel: w379 -> [w390 _]
                      tunnel: ["不合格" "报表"] -> w378
                      frame False {
                        n326 = global read "Global.vi" "程序固化引用句柄"() -> (w392:refnum<vi>)
                        n327 = call "设备状态.vi"("枚举"=enum16{"Read", "Write"}."Write", "工位"=enum16{"工位一", "工位二"}."工位一", "Status_Write"=i16 400) -> ()  [unwired: 8 in, 1 out]
                        n328 = local read "判定结果"() -> (w385:bool[][])
                        n329 = Build Array (concatenate)(w385, bool[][] [[TRUE, FALSE]] ("判定结果")) -> (w387:bool[][])
                        n330 = Concatenate Strings("程序固化失败！\n可能的原因是：\n" ("字符串"), w390) -> (w389:string)
                        n331 = property class="检测CTR"(reference=w392, "Value"=T4."Faild" ("值")) -> ()  [unwired: 1 in, 2 out]
                        n332 = local write "判定结果"(w387) -> ()
                        n333 = One Button Dialog(message=w389) -> ()  [unwired: 1 in, 1 out]
                      }
                      frame True {
                        n334 = local read "判定结果"() -> (w397:bool[][])
                        n335 = Build Array (concatenate)(w397, bool[][] [[TRUE, TRUE]] ("判定结果")) -> (w399:bool[][])
                        n336 = global read "Global.vi" "程序固化引用句柄"() -> (w401:refnum<vi>)
                        n337 = local write "判定结果"(w399) -> ()
                        n338 = call "设备状态.vi"("枚举"=enum16{"Read", "Write"}."Write", "工位"=enum16{"工位一", "工位二"}."工位一", "Status_Write"=i16 400) -> ()  [unwired: 8 in, 1 out]
                        n339 = property class="检测CTR"(reference=w401, "Value"=T4."Pass" ("值")) -> ()  [unwired: 1 in, 2 out]
                      }
                    }
                    n340 = local write "STEP"(w378) -> ()
                  }
                }
              }
              frame True {
                n341 = call "设备状态.vi"("枚举"=enum16{"Read", "Write"}."Write", "工位"=enum16{"工位一", "工位二"}."工位一", "Status_Write"=i16 400) -> ()  [unwired: 8 in, 1 out]
                n342 = local read "判定结果"() -> (w407:bool[][])
                n343 = local write "STEP"("报表" ("STEP")) -> ()
                n344 = Build Array (concatenate)(w407, bool[][] [[FALSE, FALSE]] ("判定结果")) -> (w409:bool[][])
                n345 = local write "判定结果"(w409) -> ()
              }
            }
          }
          frame "程序复检" {
            n346 = global read "Global.vi" "传感器特性用句柄"() -> (w414:refnum<vi>)
            n347 = property class="检测CTR"(reference=w414) -> ("Value"=w415:variant)  [unwired: 1 in, 2 out]
            n348 = Variant To Data(type=检测CTR数据."Idle" ("Data"), Variant=w415) -> (data=w413:T2)  [unwired: 1 in, 1 out]
            n349 = Equal?(x=w413, y=检测CTR数据."Skip" ("Data")) -> (x = y?=w410:bool)
            n350 = case shown="真" w410 {
              frame False {
                n351 = stacked-sequence {
                  frame #0 {
                    n352 = global read "Global.vi" "传感器特性用句柄"() -> (w418:refnum<vi>)
                    n353 = call "浮动通知.vi"("通知内容"="传感器特性" ("Status")) -> ()  [unwired: 11 in]
                    n354 = property class="检测CTR"(reference=w418, "Value"=T4."Runing" ("值")) -> ()  [unwired: 1 in, 2 out]
                    n355 = for {
                      tunnel: string[] ["PS采集.vi"] -> [w420] mode=indexing
                      n356 = call "CloseVI.vi"("名称或相对路径"=w420) -> ()  [unwired: 10 in, 1 out]
                    }
                  }
                  frame #1 {
                    n357 = vi-ref "T1T2占空比.vi"() -> (w422:refnum<vi>)
                    n358 = call "CallVI.vi"("VI引用"=w422, "状态"=T3."Hidden") -> ()  [unwired: 12 in, 2 out]
                    n359 = local write "STEP"("自动" ("STEP")) -> ()
                    n360 = call "设备状态.vi"("枚举"=enum16{"Read", "Write"}."Write", "工位"=enum16{"工位一", "工位二"}."工位一", "Status_Write"=i16 300) -> ()  [unwired: 8 in, 1 out]
                  }
                  frame #2 {
                    n361 = vi-ref "扭矩.vi"() -> (w428:refnum<vi>)
                    n362 = call "CallVI.vi"("VI引用"=w428, "状态"=T3."Hidden") -> ()  [unwired: 12 in, 2 out]
                  }
                }
              }
              frame True {
                n363 = flat-sequence {
                  frame #0 {
                    n364 = local read "判定结果"() -> (w429:bool[][])
                    n365 = Build Array (concatenate)(w429, bool[][] [[FALSE, TRUE]] ("判定结果")) -> (w431:bool[][])
                    n366 = local write "判定结果"(w431) -> ()
                  }
                  frame #1 {
                    n367 = local write "STEP"("程序固化" ("STEP")) -> ()
                  }
                }
              }
            }
          }
          frame "复检判定" {
            n368 = global read "Global.vi" "复检判定参数"() -> (w443:T8)
            n369 = local read "传感器特性"() -> (w444:cluster{dbl[], dbl[]}[])
            n370 = global read "Global.vi" "Result"() -> (w445:refnum<vi>)
            n371 = global read "Global.vi" "传感器特性用句柄"() -> (w442:refnum<vi>)
            n372 = call "对中台复检判定.vi"("Result"=w445, "判定参数"=w443, "XY曲线"=w444) -> ("OK？"=w433:bool)  [unwired: 8 in]
            n373 = Select(t=T4."Pass" ("值"), s=w433, f=T4."Faild" ("值")) -> (s? t:f=w439:T4)
            n374 = Build Array(TRUE ("元素"), w433) -> (w435:bool[])
            n375 = local read "判定结果"() -> (w437:bool[][])
            n376 = property class="检测CTR"(reference=w442, "Value"=w439) -> ()  [unwired: 1 in, 2 out]
            n377 = Build Array(w435) -> (w434:bool[][])
            n378 = Build Array (concatenate)(w437, w434) -> (w438:bool[][])
            n379 = case shown="真" w433 {
              frame False {
                w458 = enum16{"Read", "Write"}."Write" ("枚举")
                n380 = call "设备状态.vi"("枚举"=w458, "工位"=enum16{"工位一", "工位二"}."工位一", "Status_Write"=i16 400) -> ()  [unwired: 8 in, 1 out]
                n381 = local write "STEP"("报表" ("STEP")) -> ()
                n382 = call "合格状态.vi"("枚举"=w458, "工位"=enum16{"工位一", "工位二"}."工位一", "Status_Write"=i16 2) -> ()  [unwired: 8 in, 1 out]
              }
              frame True {
                n383 = local write "STEP"("程序固化" ("STEP")) -> ()
              }
            }
            n384 = local write "判定结果"(w438) -> ()
            n385 = disable-structure shown="禁用" {
              frame Disabled {
                n386 = Two Button Dialog(message="复检失败\n请选择是否继续？" ("消息"), 1:"否" ("F按钮名称（“取消”）"), 2:"是" ("T按钮名称（“确定”）")) -> (T button?=w449:bool)
                n387 = case shown="假" w449 {
                  tunnel: ["报表" ("STEP") "程序固化" ("STEP")] -> w450
                  frame False {
                    n388 = call "设备状态.vi"("枚举"=enum16{"Read", "Write"}."Write", "工位"=enum16{"工位一", "工位二"}."工位一", "Status_Write"=i16 400) -> ()  [unwired: 8 in, 1 out]
                  }
                  frame True {
                  }
                }
                n389 = local write "STEP"(w450) -> ()
              }
              frame Enabled {
              }
            }
          }
          frame "自动" {
            n390 = global read "Global.vi" "产品型号"() -> (w463:string)
            n391 = call "设备状态.vi"("工位"=enum16{"工位一", "工位二"}."工位一") -> ("Status_Read"=w465:i16)  [unwired: 10 in]
            n392 = case shown="401" w465 {
              tunnel: w463 -> [_ _ _ _ _ w474 _ _ _ _ _ _ _ _ w913 _ _ _ _ _ _ _ _ _ _ _ _ _ _]
              frame -128 {
                n393 = global write "Global.vi" "计时开始"(FALSE ("计时开始")) -> ()
                n394 = call "浮动通知.vi"("通知内容"="复位中……" ("Status")) -> ()  [unwired: 11 in]
              }
              frame 0, Default {
              }
              frame 1 {
                n395 = call "浮动通知.vi"("通知内容"="请复位！" ("Status")) -> ()  [unwired: 11 in]
              }
              frame 5 {
                n396 = global write "Global.vi" "计时开始"(FALSE ("计时开始")) -> ()
                n397 = call "浮动通知.vi"("通知内容"="复位完成" ("Status")) -> ()  [unwired: 11 in]
              }
              frame 8 {
                n398 = call "浮动通知.vi"("通知内容"="程序停止！" ("Status")) -> ()  [unwired: 11 in]
              }
              frame 10 {
                n399 = case shown="默认" w474 {
                  tunnel: [_ "扫码" ("STEP") "扫码" ("STEP") "传感器码" ("STEP") "传感器码" ("STEP") "传感器码" ("STEP") "传感器码" ("STEP") "传感器码" ("STEP")] -> w472
                  frame Default {
                  }
                  frame "R128" {
                  }
                  frame "R567X" {
                  }
                  frame "R092B" {
                  }
                  frame "R128K" {
                  }
                  frame "R128G" {
                  }
                  frame "R128H" {
                  }
                  frame "R563X" {
                  }
                }
                n400 = Wait Until Next ms Multiple(millisecond multiple=u32 50 ("等待时间（毫秒）")) -> ()  [unwired: 1 out]
                n401 = local write "STEP"(w472) -> ()
              }
              frame 300 {
                n402 = call "设备状态.vi"("枚举"=enum16{"Read", "Write"}."Write", "工位"=enum16{"工位一", "工位二"}."工位一", "Status_Write"=i16 310) -> ()  [unwired: 8 in, 1 out]
              }
              frame 310 {
                n403 = global read "Global.vi" "扭矩"() -> (w500:cluster{"工位一":dbl, "工位二":dbl})
                n404 = call "传感器数据.vi"() -> ("传感器读数"=w491:T6)  [unwired: 11 in]
                n405 = global read "Global.vi" "工位一扭矩"() -> (w487:dbl)
                n406 = global read "excursion.vi" "excursion"() -> (w489:T7)
                n407 = Unbundle By Name(w491) -> ("工位一驱动伺服位移"=w492:sgl)
                n408 = global read "Global.vi" "复检参数"() -> (w486:T9)
                n409 = Unbundle By Name(w500) -> ()  [unwired: 1 out]
                n410 = global read "Global.vi" "保护角度"() -> (w496:dbl)
                n411 = local read "初始角度"() -> (w493:dbl)
                n412 = Unbundle By Name(w489) -> ("左逆向"=w488:dbl)
                n413 = Unbundle By Name(w486) -> ()  [unwired: 1 out]
                n414 = Subtract(x=w492, y=w493) -> (x-y=w494:dbl)
                n415 = Subtract(x=w487, y=w488) -> (x-y=w499:dbl)
                n416 = Absolute Value(x=w494) -> (abs(x)=w495:dbl)
                n417 = Less Or Equal?(x=w499, y=-6.0) -> (x <= y?=w498:bool)
                n418 = Greater Or Equal?(x=w495, y=w496) -> (x >= y?=w490:bool)
                n419 = Compound Arithmetic op=OR ("复合运算")(w498, w490) -> (w497:bool)
                n420 = case shown="真" w497 {
                  tunnel: w487 -> [w502 _]
                  tunnel: w490 -> [_ w523]
                  frame False {
                    n421 = feedback #1() -> (w518:dbl)  [unwired: 1 in]
                    n422 = feedback-in #1(w502) -> ()
                    n423 = feedback #2() -> (w510:dbl)  [unwired: 1 in]
                    n424 = Equal?(x=w502, y=w518) -> (x = y?=w516:bool)
                    n425 = feedback #3() -> (w517:dbl)  [unwired: 1 in]
                    n426 = feedback-in #3(w518) -> ()
                    n427 = feedback #4() -> (w509:dbl)  [unwired: 1 in]
                    n428 = feedback-in #4(w510) -> ()
                    n429 = Equal?(x=w502, y=w510) -> (x = y?=w507:bool)
                    n430 = feedback #5() -> (w508:dbl)  [unwired: 1 in]
                    n431 = feedback-in #5(w509) -> ()
                    n432 = Equal?(x=w502, y=w517) -> (x = y?=w515:bool)
                    n433 = Equal?(x=w502, y=w509) -> (x = y?=w506:bool)
                    n434 = feedback #6() -> (w513:dbl)  [unwired: 1 in]
                    n435 = feedback-in #6(w517) -> ()
                    n436 = feedback #7() -> (w503:dbl)  [unwired: 1 in]
                    n437 = feedback-in #7(w508) -> ()
                    n438 = Equal?(x=w502, y=w513) -> (x = y?=w514:bool)
                    n439 = feedback #8() -> (w511:dbl)  [unwired: 1 in]
                    n440 = feedback-in #2(w511) -> ()
                    n441 = feedback-in #8(w513) -> ()
                    n442 = Equal?(x=w502, y=w508) -> (x = y?=w505:bool)
                    n443 = Equal?(x=w502, y=w511) -> (x = y?=w512:bool)
                    n444 = Equal?(x=w502, y=w503) -> (x = y?=w504:bool)
                    n445 = Compound Arithmetic op=AND(w516, w515, w514, w512, w507, w506, w505, w504) -> ()  [unwired: 1 out]
                    n446 = case shown="假" FALSE {
                      frame False {
                      }
                      frame True {
                        n447 = call "设备状态.vi"("枚举"=enum16{"Read", "Write"}."Write", "工位"=enum16{"工位一", "工位二"}."工位一", "Status_Write"=i16 316) -> ()  [unwired: 8 in, 1 out]
                        n448 = One Button Dialog(message="角度采集异常！\n请重启应用程序！" ("消息")) -> ()  [unwired: 1 in, 1 out]
                      }
                    }
                  }
                  frame True {
                    n449 = case shown="假" w523 {
                      frame False {
                        n450 = flat-sequence {
                          frame #0 {
                            n451 = call "工位暂停.vi"("枚举"=enum16{"Read", "Write"}."Write", "工位"=enum16{"工位一", "工位二"}."工位一", "Status_Write"=i16 1) -> ()  [unwired: 8 in, 1 out]
                            n452 = call "设备状态.vi"("枚举"=enum16{"Read", "Write"}."Write", "工位"=enum16{"工位一", "工位二"}."工位一", "Status_Write"=i16 311) -> ()  [unwired: 8 in, 1 out]
                          }
                          frame #1 {
                            n453 = Wait (ms)(milliseconds to wait=u32 300 ("等待时间（毫秒）")) -> ()  [unwired: 1 out]
                          }
                        }
                      }
                      frame True {
                        n454 = call "设备状态.vi"("枚举"=enum16{"Read", "Write"}."Write", "工位"=enum16{"工位一", "工位二"}."工位一", "Status_Write"=i16 316) -> ()  [unwired: 8 in, 1 out]
                        n455 = One Button Dialog(message="扭矩采集异常！\n请重启应用程序！" ("消息")) -> ()  [unwired: 1 in, 1 out]
                      }
                    }
                  }
                }
              }
              frame 311 {
                n456 = global read "Global.vi" "扭矩"() -> (w541:cluster{"工位一":dbl, "工位二":dbl})
                n457 = global read "excursion.vi" "excursion"() -> (w539:T7)
                n458 = global read "Global.vi" "工位一扭矩"() -> (w535:dbl)
                n459 = Unbundle By Name(w541) -> ()  [unwired: 1 out]
                n460 = Unbundle By Name(w539) -> ("左正向"=w538:dbl)
                n461 = Subtract(x=w535, y=w538) -> (x-y=w537:dbl)
                n462 = Greater Or Equal?(x=w537, y=0.0) -> (x >= y?=w540:bool)
                n463 = case shown="真" w540 {
                  frame False {
                    n464 = call "工位暂停.vi"("枚举"=enum16{"Read", "Write"}."Write", "工位"=enum16{"工位一", "工位二"}."工位一", "Status_Write"=i16 0) -> ()  [unwired: 8 in, 1 out]
                  }
                  frame True {
                    n465 = flat-sequence {
                      frame #0 {
                        n466 = call "设备状态.vi"("枚举"=enum16{"Read", "Write"}."Write", "工位"=enum16{"工位一", "工位二"}."工位一", "Status_Write"=i16 312) -> ()  [unwired: 8 in, 1 out]
                        n467 = call "工位暂停.vi"("枚举"=enum16{"Read", "Write"}."Write", "工位"=enum16{"工位一", "工位二"}."工位一", "Status_Write"=i16 1) -> ()  [unwired: 8 in, 1 out]
                      }
                      frame #1 {
                        n468 = Wait (ms)(milliseconds to wait=u32 500 ("等待时间（毫秒）")) -> ()  [unwired: 1 out]
                      }
                    }
                  }
                }
              }
              frame 312 {
                n469 = call "传感器数据.vi"() -> ("传感器读数"=w556:T6)  [unwired: 11 in]
                n470 = global read "excursion.vi" "excursion"() -> (w554:T7)
                n471 = global read "Global.vi" "扭矩"() -> (w567:cluster{"工位一":dbl, "工位二":dbl})
                n472 = Unbundle By Name(w556) -> ("工位一驱动伺服位移"=w557:sgl)
                n473 = global read "Global.vi" "工位一扭矩"() -> (w552:dbl)
                n474 = Unbundle By Name(w567) -> ()  [unwired: 1 out]
                n475 = global read "Global.vi" "复检参数"() -> (w566:T9)
                n476 = global read "Global.vi" "保护角度"() -> (w561:dbl)
                n477 = local read "初始角度"() -> (w558:dbl)
                n478 = Unbundle By Name(w554) -> ("右上升"=w553:dbl)
                n479 = Unbundle By Name(w566) -> ("换向扭矩"=w565:dbl)
                n480 = Subtract(x=w557, y=w558) -> (x-y=w559:dbl)
                n481 = Subtract(x=w552, y=w553) -> (x-y=w563:dbl)
                n482 = Absolute Value(x=w559) -> (abs(x)=w560:dbl)
                n483 = Greater Or Equal?(x=w560, y=w561) -> (x >= y?=w555:bool)
                n484 = Greater Or Equal?(x=w563, y=w565) -> (x >= y?=w564:bool)
                n485 = Compound Arithmetic op=OR ("复合运算")(w564, w555) -> (w562:bool)
                n486 = case shown="假" w562 {
                  tunnel: w563 -> [w573 _]
                  tunnel: w555 -> [_ w630]
                  frame False {
                    n487 = local read "传感器特性"() -> (w574:cluster{dbl[], dbl[]}[])
                    n488 = local read "初始化"() -> (w572:bool[])
                    n489 = for {
                      tunnel: w574 -> [w582] mode=indexing
                      tunnel: [w581] -> w575 mode=indexing
                      tunnel: w573 -> [w580]
                      tunnel: w572 -> [w579] mode=indexing
                      tunnel: [w578] -> w571 mode=indexing
                      i -> [w583]
                      n490 = case shown="0" w583 {
                        tunnel: w582 -> [w585 w596 w610 w626]
                        tunnel: [w585 w594 w608 w622] -> w581
                        tunnel: w580 -> [_ w587 w601 w615]
                        tunnel: w579 -> [w584 w591 w602 w617]
                        tunnel: [w584 FALSE ("布尔") FALSE ("布尔") FALSE ("布尔")] -> w578
                        tunnel: 2 -> [_ w590 w606 w616]
                        tunnel: 2 -> [_ w589 w604 w618]
                        frame Default {
                        }
                        frame 0 {
                          n491 = global read "Global.vi" "工位一T1"() -> (w592:dbl)
                          n492 = Unbundle(w596) -> (w599:dbl[], w595:dbl[])
                          n493 = call-poly <userlib>:"MGI Running Average.vi"("Averaging Size"=w590, "Initialize? (F)"=w591, "Value"=w587) -> ("Average"=w586:dbl)  [unwired: 8 in]
                          n494 = call-poly <userlib>:"MGI Running Average.vi"("Averaging Size"=w589, "Initialize? (F)"=w591, "Value"=w592) -> ("Average"=w588:dbl)  [unwired: 8 in]
                          n495 = Build Array (concatenate)(w599, w586) -> (w598:dbl[])
                          n496 = Build Array (concatenate)(w595, w588) -> (w597:dbl[])
                          n497 = Bundle(w598, w597) -> (w594:cluster{dbl[], dbl[]})  [unwired: 1 in]
                        }
                        frame 1 {
                          n498 = global read "Global.vi" "工位一T2"() -> (w605:dbl)
                          n499 = Unbundle(w610) -> (w613:dbl[], w609:dbl[])
                          n500 = call-poly <userlib>:"MGI Running Average.vi"("Averaging Size"=w606, "Initialize? (F)"=w602, "Value"=w601) -> ("Average"=w600:dbl)  [unwired: 8 in]
                          n501 = call-poly <userlib>:"MGI Running Average.vi"("Averaging Size"=w604, "Initialize? (F)"=w602, "Value"=w605) -> ("Average"=w603:dbl)  [unwired: 8 in]
                          n502 = Build Array (concatenate)(w609, w603) -> (w611:dbl[])
                          n503 = Build Array (concatenate)(w613, w600) -> (w612:dbl[])
                          n504 = Bundle(w612, w611) -> (w608:cluster{dbl[], dbl[]})  [unwired: 1 in]
                        }
                        frame 2 {
                          n505 = Unbundle(w626) -> (w629:dbl[], w625:dbl[])
                          n506 = global read "Global.vi" "工位一T1"() -> (w624:dbl)
                          n507 = global read "Global.vi" "工位一T2"() -> (w623:dbl)
                          n508 = call-poly <userlib>:"MGI Running Average.vi"("Averaging Size"=w616, "Initialize? (F)"=w617, "Value"=w615) -> ("Average"=w614:dbl)  [unwired: 8 in]
                          n509 = Add(x=w624, y=w623) -> (x+y=w620:dbl)
                          n510 = call-poly <userlib>:"MGI Running Average.vi"("Averaging Size"=w618, "Initialize? (F)"=w617, "Value"=w620) -> ("Average"=w619:dbl)  [unwired: 8 in]
                          n511 = Build Array (concatenate)(w629, w614) -> (w628:dbl[])
                          n512 = Build Array (concatenate)(w625, w619) -> (w627:dbl[])
                          n513 = Bundle(w628, w627) -> (w622:cluster{dbl[], dbl[]})  [unwired: 1 in]
                        }
                      }
                    }
                    n514 = call "工位暂停.vi"("枚举"=enum16{"Read", "Write"}."Write", "工位"=enum16{"工位一", "工位二"}."工位一", "Status_Write"=i16 0) -> ()  [unwired: 8 in, 1 out]
                    n515 = local write "初始化"(w571) -> ()
                    n516 = local write "传感器特性"(w575) -> ()
                  }
                  frame True {
                    n517 = case shown="假" w630 {
                      frame False {
                        n518 = flat-sequence {
                          frame #0 {
                            n519 = call "工位暂停.vi"("枚举"=enum16{"Read", "Write"}."Write", "工位"=enum16{"工位一", "工位二"}."工位一", "Status_Write"=i16 1) -> ()  [unwired: 8 in, 1 out]
                            n520 = call "设备状态.vi"("枚举"=enum16{"Read", "Write"}."Write", "工位"=enum16{"工位一", "工位二"}."工位一", "Status_Write"=i16 313) -> ()  [unwired: 8 in, 1 out]
                          }
                          frame #1 {
                            n521 = Wait (ms)(milliseconds to wait=u32 500 ("等待时间（毫秒）")) -> ()  [unwired: 1 out]
                          }
                        }
                      }
                      frame True {
                        n522 = call "设备状态.vi"("枚举"=enum16{"Read", "Write"}."Write", "工位"=enum16{"工位一", "工位二"}."工位一", "Status_Write"=i16 316) -> ()  [unwired: 8 in, 1 out]
                        n523 = One Button Dialog(message="扭矩采集异常！\n请重启应用程序！" ("消息")) -> ()  [unwired: 1 in, 1 out]
                      }
                    }
                  }
                }
              }
              frame 313 {
                n524 = call "传感器数据.vi"() -> ("传感器读数"=w652:T6)  [unwired: 11 in]
                n525 = global read "Global.vi" "复检参数"() -> (w657:T9)
                n526 = global read "excursion.vi" "excursion"() -> (w655:T7)
                n527 = Unbundle By Name(w652) -> ("工位一驱动伺服位移"=w651:sgl)
                n528 = global read "Global.vi" "扭矩"() -> (w658:cluster{"工位一":dbl, "工位二":dbl})
                n529 = global read "Global.vi" "保护角度"() -> (w647:dbl)
                n530 = local read "初始角度"() -> (w650:dbl)
                n531 = global read "Global.vi" "工位一扭矩"() -> (w644:dbl)
                n532 = Unbundle By Name(w657) -> ("换向扭矩"=w656:dbl)
                n533 = Unbundle By Name(w658) -> ()  [unwired: 1 out]
                n534 = Unbundle By Name(w655) -> ("右下降"=w653:dbl)
                n535 = Subtract(x=w651, y=w650) -> (x-y=w649:dbl)
                n536 = Absolute Value(x=w649) -> (abs(x)=w648:dbl)
                n537 = Subtract(x=w644, y=w653) -> (x-y=w645:dbl)
                n538 = Greater Or Equal?(x=w648, y=w647) -> (x >= y?=w646:bool)
                n539 = Less?(x=w645, y=0.0) -> (x < y?=w642:bool)
                n540 = Less Or Equal?(x=w645, y=w656) -> (x <= y?=w643:bool)
                n541 = case shown="假" w642 {
                  tunnel: w645 -> [w664 _]
                  tunnel: w643 -> [w659 _]
                  tunnel: w646 -> [w660 _]
                  frame False {
                    n542 = case shown="真" w659 {
                      tunnel: w664 -> [_ w668]
                      tunnel: w660 -> [w665 _]
                      frame False {
                        n543 = case shown="真" w665 {
                          frame False {
                          }
                          frame True {
                          }
                        }
                      }
                      frame True {
                        n544 = local read "传感器特性"() -> (w669:cluster{dbl[], dbl[]}[])
                        n545 = local read "初始化"() -> (w667:bool[])
                        n546 = for {
                          tunnel: w669 -> [w677] mode=indexing
                          tunnel: [w676] -> w670 mode=indexing
                          tunnel: w668 -> [w675]
                          tunnel: w667 -> [w674] mode=indexing
                          tunnel: [w673] -> w666 mode=indexing
                          i -> [w678]
                          n547 = case shown="5" w678 {
                            tunnel: w677 -> [w680 w691 w705 w721]
                            tunnel: [w680 w689 w703 w717] -> w676
                            tunnel: w675 -> [_ w682 w696 w710]
                            tunnel: w674 -> [w679 w686 w698 w714]
                            tunnel: [w679 FALSE ("布尔") FALSE ("布尔") FALSE ("布尔")] -> w673
                            tunnel: 2 -> [_ w685 w697 w713]
                            tunnel: 2 -> [_ w684 w700 w711]
                            frame Default {
                            }
                            frame 3 {
                              n548 = global read "Global.vi" "工位一T1"() -> (w687:dbl)
                              n549 = Unbundle(w691) -> (w694:dbl[], w690:dbl[])
                              n550 = call-poly <userlib>:"MGI Running Average.vi"("Averaging Size"=w685, "Initialize? (F)"=w686, "Value"=w682) -> ("Average"=w681:dbl)  [unwired: 8 in]
                              n551 = call-poly <userlib>:"MGI Running Average.vi"("Averaging Size"=w684, "Initialize? (F)"=w686, "Value"=w687) -> ("Average"=w683:dbl)  [unwired: 8 in]
                              n552 = Build Array (concatenate)(w694, w681) -> (w693:dbl[])
                              n553 = Build Array (concatenate)(w690, w683) -> (w692:dbl[])
                              n554 = Bundle(w693, w692) -> (w689:cluster{dbl[], dbl[]})  [unwired: 1 in]
                            }
                            frame 4 {
                              n555 = global read "Global.vi" "工位一T2"() -> (w701:dbl)
                              n556 = Unbundle(w705) -> (w708:dbl[], w704:dbl[])
                              n557 = call-poly <userlib>:"MGI Running Average.vi"("Averaging Size"=w697, "Initialize? (F)"=w698, "Value"=w696) -> ("Average"=w695:dbl)  [unwired: 8 in]
                              n558 = call-poly <userlib>:"MGI Running Average.vi"("Averaging Size"=w700, "Initialize? (F)"=w698, "Value"=w701) -> ("Average"=w699:dbl)  [unwired: 8 in]
                              n559 = Build Array (concatenate)(w704, w699) -> (w706:dbl[])
                              n560 = Build Array (concatenate)(w708, w695) -> (w707:dbl[])
                              n561 = Bundle(w707, w706) -> (w703:cluster{dbl[], dbl[]})  [unwired: 1 in]
                            }
                            frame 5 {
                              n562 = Unbundle(w721) -> (w724:dbl[], w720:dbl[])
                              n563 = global read "Global.vi" "工位一T1"() -> (w719:dbl)
                              n564 = global read "Global.vi" "工位一T2"() -> (w718:dbl)
                              n565 = call-poly <userlib>:"MGI Running Average.vi"("Averaging Size"=w713, "Initialize? (F)"=w714, "Value"=w710) -> ("Average"=w709:dbl)  [unwired: 8 in]
                              n566 = Add(x=w719, y=w718) -> (x+y=w715:dbl)
                              n567 = call-poly <userlib>:"MGI Running Average.vi"("Averaging Size"=w711, "Initialize? (F)"=w714, "Value"=w715) -> ("Average"=w712:dbl)  [unwired: 8 in]
                              n568 = Build Array (concatenate)(w724, w709) -> (w723:dbl[])
                              n569 = Build Array (concatenate)(w720, w712) -> (w722:dbl[])
                              n570 = Bundle(w723, w722) -> (w717:cluster{dbl[], dbl[]})  [unwired: 1 in]
                            }
                          }
                        }
                        n571 = local write "初始化"(w666) -> ()
                        n572 = local write "传感器特性"(w670) -> ()
                      }
                    }
                    n573 = call "工位暂停.vi"("枚举"=enum16{"Read", "Write"}."Write", "工位"=enum16{"工位一", "工位二"}."工位一", "Status_Write"=i16 0) -> ()  [unwired: 8 in, 1 out]
                  }
                  frame True {
                    n574 = flat-sequence {
                      frame #0 {
                        n575 = call "设备状态.vi"("枚举"=enum16{"Read", "Write"}."Write", "工位"=enum16{"工位一", "工位二"}."工位一", "Status_Write"=i16 314) -> ()  [unwired: 8 in, 1 out]
                        n576 = call "工位暂停.vi"("枚举"=enum16{"Read", "Write"}."Write", "工位"=enum16{"工位一", "工位二"}."工位一", "Status_Write"=i16 1) -> ()  [unwired: 8 in, 1 out]
                      }
                      frame #1 {
                        n577 = Wait (ms)(milliseconds to wait=u32 500 ("等待时间（毫秒）")) -> ()  [unwired: 1 out]
                      }
                    }
                  }
                }
              }
              frame 314 {
                n578 = global read "excursion.vi" "excursion"() -> (w734:T7)
                n579 = call "传感器数据.vi"() -> ("传感器读数"=w737:T6)  [unwired: 11 in]
                n580 = global read "Global.vi" "复检参数"() -> (w746:T9)
                n581 = global read "Global.vi" "扭矩"() -> (w747:cluster{"工位一":dbl, "工位二":dbl})
                n582 = Unbundle By Name(w737) -> ("工位一驱动伺服位移"=w738:sgl)
                n583 = global read "Global.vi" "工位一扭矩"() -> (w732:dbl)
                n584 = global read "Global.vi" "保护角度"() -> (w742:dbl)
                n585 = Unbundle By Name(w747) -> ()  [unwired: 1 out]
                n586 = Unbundle By Name(w746) -> ("换向扭矩"=w745:dbl)
                n587 = local read "初始角度"() -> (w739:dbl)
                n588 = Unbundle By Name(w734) -> ("左上升"=w733:dbl)
                n589 = Subtract(x=w732, y=w733) -> (x-y=w743:dbl)
                n590 = Subtract(x=w738, y=w739) -> (x-y=w740:dbl)
                n591 = Negate(x=w745) -> (-x=w748:dbl)
                n592 = Absolute Value(x=w740) -> (abs(x)=w741:dbl)
                n593 = Less Or Equal?(x=w743, y=w748) -> (x <= y?=w744:bool)
                n594 = Greater Or Equal?(x=w741, y=w742) -> (x >= y?=w735:bool)
                n595 = Compound Arithmetic op=OR ("复合运算")(w744, w735) -> (w736:bool)
                n596 = case shown="假" w736 {
                  tunnel: w743 -> [w754 _]
                  tunnel: w743 -> [w753 _]
                  tunnel: w735 -> [_ w814]
                  frame False {
                    n597 = Less Or Equal To 0?(x=w753) -> (x <= 0?=w752:bool)
                    n598 = case shown="真" w752 {
                      tunnel: w754 -> [_ w759]
                      frame False {
                      }
                      frame True {
                        n599 = local read "传感器特性"() -> (w757:cluster{dbl[], dbl[]}[])
                        n600 = local read "初始化"() -> (w756:bool[])
                        n601 = for {
                          tunnel: w757 -> [w766] mode=indexing
                          tunnel: [w765] -> w758 mode=indexing
                          tunnel: w759 -> [w764]
                          tunnel: w756 -> [w763] mode=indexing
                          tunnel: [w762] -> w755 mode=indexing
                          i -> [w767]
                          n602 = case shown="7" w767 {
                            tunnel: w766 -> [w769 w780 w794 w810]
                            tunnel: [w769 w778 w792 w806] -> w765
                            tunnel: w764 -> [_ w771 w785 w799]
                            tunnel: w763 -> [w768 w773 w787 w801]
                            tunnel: [w768 FALSE ("布尔") FALSE ("布尔") FALSE ("布尔")] -> w762
                            tunnel: 2 -> [_ w775 w789 w803]
                            tunnel: 2 -> [_ w772 w786 w800]
                            frame Default {
                            }
                            frame 6 {
                              n603 = Unbundle(w780) -> (w783:dbl[], w779:dbl[])
                              n604 = global read "Global.vi" "工位一T1"() -> (w776:dbl)
                              n605 = call-poly <userlib>:"MGI Running Average.vi"("Averaging Size"=w772, "Initialize? (F)"=w773, "Value"=w771) -> ("Average"=w770:dbl)  [unwired: 8 in]
                              n606 = call-poly <userlib>:"MGI Running Average.vi"("Averaging Size"=w775, "Initialize? (F)"=w773, "Value"=w776) -> ("Average"=w774:dbl)  [unwired: 8 in]
                              n607 = Build Array (concatenate)(w779, w774) -> (w781:dbl[])
                              n608 = Build Array (concatenate)(w783, w770) -> (w782:dbl[])
                              n609 = Bundle(w782, w781) -> (w778:cluster{dbl[], dbl[]})  [unwired: 1 in]
                            }
                            frame 7 {
                              n610 = Unbundle(w794) -> (w797:dbl[], w793:dbl[])
                              n611 = global read "Global.vi" "工位一T2"() -> (w790:dbl)
                              n612 = call-poly <userlib>:"MGI Running Average.vi"("Averaging Size"=w786, "Initialize? (F)"=w787, "Value"=w785) -> ("Average"=w784:dbl)  [unwired: 8 in]
                              n613 = call-poly <userlib>:"MGI Running Average.vi"("Averaging Size"=w789, "Initialize? (F)"=w787, "Value"=w790) -> ("Average"=w788:dbl)  [unwired: 8 in]
                              n614 = Build Array (concatenate)(w797, w784) -> (w796:dbl[])
                              n615 = Build Array (concatenate)(w793, w788) -> (w795:dbl[])
                              n616 = Bundle(w796, w795) -> (w792:cluster{dbl[], dbl[]})  [unwired: 1 in]
                            }
                            frame 8 {
                              n617 = Unbundle(w810) -> (w813:dbl[], w809:dbl[])
                              n618 = global read "Global.vi" "工位一T1"() -> (w808:dbl)
                              n619 = global read "Global.vi" "工位一T2"() -> (w807:dbl)
                              n620 = call-poly <userlib>:"MGI Running Average.vi"("Averaging Size"=w800, "Initialize? (F)"=w801, "Value"=w799) -> ("Average"=w798:dbl)  [unwired: 8 in]
                              n621 = Add(x=w808, y=w807) -> (x+y=w804:dbl)
                              n622 = call-poly <userlib>:"MGI Running Average.vi"("Averaging Size"=w803, "Initialize? (F)"=w801, "Value"=w804) -> ("Average"=w802:dbl)  [unwired: 8 in]
                              n623 = Build Array (concatenate)(w809, w802) -> (w811:dbl[])
                              n624 = Build Array (concatenate)(w813, w798) -> (w812:dbl[])
                              n625 = Bundle(w812, w811) -> (w806:cluster{dbl[], dbl[]})  [unwired: 1 in]
                            }
                          }
                        }
                        n626 = local write "初始化"(w755) -> ()
                        n627 = local write "传感器特性"(w758) -> ()
                      }
                    }
                    n628 = call "工位暂停.vi"("枚举"=enum16{"Read", "Write"}."Write", "工位"=enum16{"工位一", "工位二"}."工位一", "Status_Write"=i16 0) -> ()  [unwired: 8 in, 1 out]
                  }
                  frame True {
                    n629 = case shown="假" w814 {
                      frame False {
                        n630 = flat-sequence {
                          frame #0 {
                            n631 = call "工位暂停.vi"("枚举"=enum16{"Read", "Write"}."Write", "工位"=enum16{"工位一", "工位二"}."工位一", "Status_Write"=i16 1) -> ()  [unwired: 8 in, 1 out]
                            n632 = call "设备状态.vi"("枚举"=enum16{"Read", "Write"}."Write", "工位"=enum16{"工位一", "工位二"}."工位一", "Status_Write"=i16 315) -> ()  [unwired: 8 in, 1 out]
                          }
                          frame #1 {
                            n633 = Wait (ms)(milliseconds to wait=u32 300 ("等待时间（毫秒）")) -> ()  [unwired: 1 out]
                          }
                        }
                      }
                      frame True {
                        n634 = call "设备状态.vi"("枚举"=enum16{"Read", "Write"}."Write", "工位"=enum16{"工位一", "工位二"}."工位一", "Status_Write"=i16 316) -> ()  [unwired: 8 in, 1 out]
                        n635 = One Button Dialog(message="扭矩采集异常！\n请重启应用程序！" ("消息")) -> ()  [unwired: 1 in, 1 out]
                      }
                    }
                  }
                }
              }
              frame 315 {
                n636 = global read "excursion.vi" "excursion"() -> (w831:T7)
                n637 = global read "Global.vi" "复检参数"() -> (w833:T9)
                n638 = global read "Global.vi" "扭矩"() -> (w835:cluster{"工位一":dbl, "工位二":dbl})
                n639 = Unbundle By Name(w833) -> ("换向扭矩"=w827:dbl)
                n640 = Unbundle By Name(w831) -> ("左下降"=w830:dbl)
                n641 = Unbundle By Name(w835) -> ()  [unwired: 1 out]
                n642 = global read "Global.vi" "工位一扭矩"() -> (w829:dbl)
                n643 = Subtract(x=w829, y=w830) -> (x-y=w832:dbl)
                n644 = Negate(x=w827) -> (-x=w828:dbl)
                n645 = Greater?(x=w832, y=0.0) -> (0:w834:bool)
                n646 = case shown="假" w834 {
                  tunnel: w832 -> [w842 _]
                  tunnel: w828 -> [w841 _]
                  tunnel: w832 -> [w840 _]
                  frame False {
                    n647 = Greater Or Equal?(x=w840, y=w841) -> (x >= y?=w839:bool)
                    n648 = case shown="真" w839 {
                      tunnel: w842 -> [_ w847]
                      frame False {
                      }
                      frame True {
                        n649 = local read "传感器特性"() -> (w845:cluster{dbl[], dbl[]}[])
                        n650 = local read "初始化"() -> (w844:bool[])
                        n651 = for {
                          tunnel: w845 -> [w854] mode=indexing
                          tunnel: [w853] -> w846 mode=indexing
                          tunnel: w847 -> [w852]
                          tunnel: w844 -> [w851] mode=indexing
                          tunnel: [w850] -> w843 mode=indexing
                          i -> [w855]
                          n652 = case shown="11" w855 {
                            tunnel: w854 -> [w857 w868 w882 w898]
                            tunnel: [w857 w866 w880 w894] -> w853
                            tunnel: w852 -> [_ w859 w873 w887]
                            tunnel: w851 -> [w856 w861 w876 w891]
                            tunnel: [w856 FALSE ("布尔") FALSE ("布尔") FALSE ("布尔")] -> w850
                            tunnel: 2 -> [_ w862 w874 w888]
                            tunnel: 2 -> [_ w860 w878 w890]
                            frame Default {
                            }
                            frame 9 {
                              n653 = Unbundle(w868) -> (w871:dbl[], w867:dbl[])
                              n654 = global read "Global.vi" "工位一T1"() -> (w864:dbl)
                              n655 = call-poly <userlib>:"MGI Running Average.vi"("Averaging Size"=w860, "Initialize? (F)"=w861, "Value"=w859) -> ("Average"=w858:dbl)  [unwired: 8 in]
                              n656 = call-poly <userlib>:"MGI Running Average.vi"("Averaging Size"=w862, "Initialize? (F)"=w861, "Value"=w864) -> ("Average"=w863:dbl)  [unwired: 8 in]
                              n657 = Build Array (concatenate)(w871, w858) -> (w870:dbl[])
                              n658 = Build Array (concatenate)(w867, w863) -> (w869:dbl[])
                              n659 = Bundle(w870, w869) -> (w866:cluster{dbl[], dbl[]})  [unwired: 1 in]
                            }
                            frame 10 {
                              n660 = Unbundle(w882) -> (w885:dbl[], w881:dbl[])
                              n661 = global read "Global.vi" "工位一T2"() -> (w877:dbl)
                              n662 = call-poly <userlib>:"MGI Running Average.vi"("Averaging Size"=w878, "Initialize? (F)"=w876, "Value"=w873) -> ("Average"=w872:dbl)  [unwired: 8 in]
                              n663 = call-poly <userlib>:"MGI Running Average.vi"("Averaging Size"=w874, "Initialize? (F)"=w876, "Value"=w877) -> ("Average"=w875:dbl)  [unwired: 8 in]
                              n664 = Build Array (concatenate)(w885, w872) -> (w884:dbl[])
                              n665 = Build Array (concatenate)(w881, w875) -> (w883:dbl[])
                              n666 = Bundle(w884, w883) -> (w880:cluster{dbl[], dbl[]})  [unwired: 1 in]
                            }
                            frame 11 {
                              n667 = Unbundle(w898) -> (w901:dbl[], w897:dbl[])
                              n668 = global read "Global.vi" "工位一T1"() -> (w896:dbl)
                              n669 = global read "Global.vi" "工位一T2"() -> (w895:dbl)
                              n670 = call-poly <userlib>:"MGI Running Average.vi"("Averaging Size"=w890, "Initialize? (F)"=w891, "Value"=w887) -> ("Average"=w886:dbl)  [unwired: 8 in]
                              n671 = Add(x=w896, y=w895) -> (x+y=w892:dbl)
                              n672 = call-poly <userlib>:"MGI Running Average.vi"("Averaging Size"=w888, "Initialize? (F)"=w891, "Value"=w892) -> ("Average"=w889:dbl)  [unwired: 8 in]
                              n673 = Build Array (concatenate)(w901, w886) -> (w900:dbl[])
                              n674 = Build Array (concatenate)(w897, w889) -> (w899:dbl[])
                              n675 = Bundle(w900, w899) -> (w894:cluster{dbl[], dbl[]})  [unwired: 1 in]
                            }
                          }
                        }
                        n676 = local write "初始化"(w843) -> ()
                        n677 = local write "传感器特性"(w846) -> ()
                      }
                    }
                    n678 = call "工位暂停.vi"("枚举"=enum16{"Read", "Write"}."Write", "工位"=enum16{"工位一", "工位二"}."工位一", "Status_Write"=i16 0) -> ()  [unwired: 8 in, 1 out]
                  }
                  frame True {
                    n679 = call "工位暂停.vi"("枚举"=enum16{"Read", "Write"}."Write", "工位"=enum16{"工位一", "工位二"}."工位一", "Status_Write"=i16 1) -> ()  [unwired: 8 in, 1 out]
                    n680 = call "设备状态.vi"("枚举"=enum16{"Read", "Write"}."Write", "工位"=enum16{"工位一", "工位二"}."工位一", "Status_Write"=i16 316) -> ()  [unwired: 8 in, 1 out]
                  }
                }
              }
              frame 316 {
                n681 = global write "Global.vi" "工位占空比采集"(FALSE ("工位二占空比采集")) -> ()
                n682 = local write "STEP"("复检判定" ("STEP")) -> ()
                n683 = call "工位暂停.vi"("枚举"=enum16{"Read", "Write"}."Write", "工位"=enum16{"工位一", "工位二"}."工位一", "Status_Write"=i16 0) -> ()  [unwired: 8 in, 1 out]
              }
              frame 401 {
                n684 = case shown="\"R567X\"" w913 {
                  frame "假", Default {
                    n685 = call "设备状态.vi"("枚举"=enum16{"Read", "Write"}."Write", "工位"=enum16{"工位一", "工位二"}."工位一", "Status_Write"=i16 10) -> ()  [unwired: 8 in, 1 out]
                  }
                  frame "R567X" {
                    n686 = local write "STEP"("程序固化" ("STEP")) -> ()
                  }
                }
              }
              frame 500 {
                n687 = global read "Global.vi" "动态优化完成"() -> (w918:bool)
                n688 = case shown="真" w918 {
                  frame False {
                    n689 = call "传感器数据.vi"() -> ("传感器读数"=w931:T6)  [unwired: 11 in]
                    n690 = Unbundle By Name(w931) -> ("工位一驱动伺服位移"=w933:sgl)
                    n691 = local read "动优化态前"() -> (w932:cluster{dbl[], dbl[]}[])
                    n692 = local read "初始化 3"() -> (w930:bool[])
                    n693 = for {
                      tunnel: [w941] -> w928 mode=indexing
                      tunnel: w933 -> [w940]
                      tunnel: w932 -> [w939] mode=indexing
                      tunnel: w930 -> [w937] mode=indexing
                      tunnel: [w936] -> w929 mode=indexing
                      i -> [w938]
                      n694 = case shown="2" w938 {
                        tunnel: [w943 w953 w965 w978 w990] -> w941
                        tunnel: w940 -> [_ w948 w960 w968 w981]
                        tunnel: w939 -> [w943 w951 w962 w975 w987]
                        tunnel: w937 -> [w942 w945 w958 w972 w984]
                        tunnel: [w942 FALSE ("布尔") FALSE ("布尔") FALSE ("布尔") FALSE ("布尔")] -> w936
                        tunnel: 15 ("rank") -> [_ _ _ w969 w983]
                        tunnel: 2 ("rank") -> [_ w944 w957 w971 _]
                        frame Default {
                        }
                        frame 0 {
                          n695 = global read "Global.vi" "工位一T1"() -> (w947:dbl)
                          n696 = call <vilib>:"Median Filter PtByPt.vi"("initialize"=w945) -> ()  [unwired: 3 in, 2 out]
                          n697 = Unbundle(w951) -> (w950:dbl[], w952:dbl[])
                          n698 = Build Array (concatenate)(w950, w948) -> (w955:dbl[])
                          n699 = call-poly <userlib>:"MGI Running Average.vi"("Averaging Size"=w944, "Initialize? (F)"=w945, "Value"=w947) -> ("Average"=w946:dbl)  [unwired: 8 in]
                          n700 = Build Array (concatenate)(w952, w946) -> (w954:dbl[])
                          n701 = Bundle(w955, w954) -> (w953:cluster{dbl[], dbl[]})  [unwired: 1 in]
                        }
                        frame 1 {
                          n702 = global read "Global.vi" "工位一T2"() -> (w959:dbl)
                          n703 = Unbundle(w962) -> (w964:dbl[], w963:dbl[])
                          n704 = call <vilib>:"Median Filter PtByPt.vi"("initialize"=w958) -> ()  [unwired: 3 in, 2 out]
                          n705 = Build Array (concatenate)(w964, w960) -> (w967:dbl[])
                          n706 = call-poly <userlib>:"MGI Running Average.vi"("Averaging Size"=w957, "Initialize? (F)"=w958, "Value"=w959) -> ("Average"=w956:dbl)  [unwired: 8 in]
                          n707 = Build Array (concatenate)(w963, w956) -> (w966:dbl[])
                          n708 = Bundle(w967, w966) -> (w965:cluster{dbl[], dbl[]})  [unwired: 1 in]
                        }
                        frame 2 {
                          n709 = global read "Global.vi" "工位一P"() -> (w973:dbl)
                          n710 = Unbundle(w975) -> (w977:dbl[], w976:dbl[])
                          n711 = call-poly <userlib>:"MGI Running Average.vi"("Averaging Size"=w971, "Initialize? (F)"=w972, "Value"=w968) -> ()  [unwired: 8 in, 1 out]
                          n712 = call-poly <userlib>:"MGI Running Average.vi"("Averaging Size"=w969, "Initialize? (F)"=w972, "Value"=w973) -> ("Average"=w970:dbl)  [unwired: 8 in]
                          n713 = Build Array (concatenate)(w977, w968) -> (w980:dbl[])
                          n714 = Build Array (concatenate)(w976, w970) -> (w979:dbl[])
                          n715 = Bundle(w980, w979) -> (w978:cluster{dbl[], dbl[]})  [unwired: 1 in]
                        }
                        frame 3 {
                          n716 = global read "Global.vi" "工位一S"() -> (w985:dbl)
                          n717 = Unbundle(w987) -> (w989:dbl[], w988:dbl[])
                          n718 = call <vilib>:"Median Filter PtByPt.vi"("initialize"=w984, "rank"=w983, "x"=w981) -> ()  [unwired: 1 in, 2 out]
                          n719 = call-poly <userlib>:"MGI Running Average.vi"("Averaging Size"=w983, "Initialize? (F)"=w984, "Value"=w985) -> ("Average"=w982:dbl)  [unwired: 8 in]
                          n720 = Build Array (concatenate)(w989, w981) -> (w992:dbl[])
                          n721 = Build Array (concatenate)(w988, w982) -> (w991:dbl[])
                          n722 = Bundle(w992, w991) -> (w990:cluster{dbl[], dbl[]})  [unwired: 1 in]
                        }
                      }
                    }
                    n723 = local write "初始化 3"(w929) -> ()
                    n724 = local write "动优化态前"(w928) -> ()
                    n725 = call "VRES值.vi"("XY"=w928, "索引1"=2, "索引2"=3) -> ("XY图 2"=w927:cluster{dbl[], dbl[]}[])  [unwired: 16 in]
                    n726 = Index Array(array=w927, index=8 ("索引")) -> (element=→"VRES_cW":cluster{dbl[], dbl[]})
                  }
                  frame True {
                    n727 = call "传感器数据.vi"() -> ("传感器读数"=w996:T6)  [unwired: 11 in]
                    n728 = Unbundle By Name(w996) -> ("工位一驱动伺服位移"=w998:sgl)
                    n729 = local read "可信度检测"() -> (w997:cluster{dbl[], dbl[]}[])
                    n730 = local read "初始化 2"() -> (w995:bool[])
                    n731 = for {
                      tunnel: [w1006] -> w993 mode=indexing
                      tunnel: w998 -> [w1005]
                      tunnel: w997 -> [w1004] mode=indexing
                      tunnel: w995 -> [w1002] mode=indexing
                      tunnel: [w1001] -> w994 mode=indexing
                      i -> [w1003]
                      n732 = case shown="2" w1003 {
                        tunnel: [w1008 w1018 w1030 w1046] -> w1006
                        tunnel: w1005 -> [_ w1013 w1025 w1038]
                        tunnel: w1004 -> [w1008 w1016 w1027 w1043]
                        tunnel: w1002 -> [w1007 w1011 w1023 w1036]
                        tunnel: [w1007 FALSE ("布尔") FALSE ("布尔") FALSE ("布尔")] -> w1001
                        tunnel: 2 ("rank") -> [_ _ _ w1039]
                        tunnel: 2 ("rank") -> [_ w1009 w1022 _]
                        frame Default {
                        }
                        frame 0 {
                          n733 = global read "Global.vi" "工位一T1"() -> (w1012:dbl)
                          n734 = Unbundle(w1016) -> (w1015:dbl[], w1017:dbl[])
                          n735 = call <vilib>:"Median Filter PtByPt.vi"("initialize"=w1011) -> ()  [unwired: 3 in, 2 out]
                          n736 = Build Array (concatenate)(w1015, w1013) -> (w1020:dbl[])
                          n737 = call-poly <userlib>:"MGI Running Average.vi"("Averaging Size"=w1009, "Initialize? (F)"=w1011, "Value"=w1012) -> ("Average"=w1010:dbl)  [unwired: 8 in]
                          n738 = Build Array (concatenate)(w1017, w1010) -> (w1019:dbl[])
                          n739 = Bundle(w1020, w1019) -> (w1018:cluster{dbl[], dbl[]})  [unwired: 1 in]
                        }
                        frame 1 {
                          n740 = global read "Global.vi" "工位一T2"() -> (w1024:dbl)
                          n741 = Unbundle(w1027) -> (w1029:dbl[], w1028:dbl[])
                          n742 = call <vilib>:"Median Filter PtByPt.vi"("initialize"=w1023) -> ()  [unwired: 3 in, 2 out]
                          n743 = Build Array (concatenate)(w1029, w1025) -> (w1032:dbl[])
                          n744 = call-poly <userlib>:"MGI Running Average.vi"("Averaging Size"=w1022, "Initialize? (F)"=w1023, "Value"=w1024) -> ("Average"=w1021:dbl)  [unwired: 8 in]
                          n745 = Build Array (concatenate)(w1028, w1021) -> (w1031:dbl[])
                          n746 = Bundle(w1032, w1031) -> (w1030:cluster{dbl[], dbl[]})  [unwired: 1 in]
                        }
                        frame 2 {
                          n747 = global read "Global.vi" "工位一P"() -> (w1040:dbl)
                          n748 = global read "Global.vi" "工位一S"() -> (w1041:dbl)
                          n749 = Unbundle(w1043) -> (w1045:dbl[], w1044:dbl[])
                          n750 = Build Array (concatenate)(w1045, w1038) -> (w1048:dbl[])
                          n751 = call "Calc_Vres.vi"("S_Data in"=w1041, "P_Data in"=w1040) -> ("Vres"=w1037:dbl)  [unwired: 7 in, 2 out]
                          n752 = call <vilib>:"Median Filter PtByPt.vi"("initialize"=w1036, "rank"=10, "x"=w1037) -> ("Filtered x"=w1034:dbl)  [unwired: 1 in, 1 out]
                          n753 = call-poly <userlib>:"MGI Running Average.vi"("Averaging Size"=w1039, "Initialize? (F)"=w1036, "Value"=w1034) -> ("Average"=w1035:dbl)  [unwired: 8 in]
                          n754 = Build Array (concatenate)(w1044, w1035) -> (w1047:dbl[])
                          n755 = Bundle(w1048, w1047) -> (w1046:cluster{dbl[], dbl[]})  [unwired: 1 in]
                        }
                      }
                    }
                    n756 = local write "初始化 2"(w994) -> ()
                    n757 = local write "可信度检测"(w993) -> ()
                  }
                }
                n758 = call "浮动通知.vi"("通知内容"="可信度检测" ("Status")) -> ()  [unwired: 11 in]
                n759 = local read "initialize 2"() -> (w921:bool)
                n760 = case shown="默认" 0 {
                  tunnel: [w1049 FALSE ("initialize 2")] -> w920
                  tunnel: w921 -> [w1049 _]
                  frame Default {
                  }
                  frame 0 {
                  }
                }
                n761 = local write "initialize 2"(w920) -> ()
              }
              frame 501 {
                n762 = global read "Global.vi" "动态优化完成"() -> (w1051:bool)
                n763 = case shown="真" w1051 {
                  frame False {
                    n764 = call "传感器数据.vi"() -> ("传感器读数"=w1064:T6)  [unwired: 11 in]
                    n765 = Unbundle By Name(w1064) -> ("工位一驱动伺服位移"=w1059:sgl)
                    n766 = local read "动优化态前"() -> (w1065:cluster{dbl[], dbl[]}[])
                    n767 = local read "初始化 3"() -> (w1063:bool[])
                    n768 = for {
                      tunnel: [w1073] -> w1060 mode=indexing
                      tunnel: w1059 -> [w1072]
                      tunnel: w1065 -> [w1071] mode=indexing
                      tunnel: w1063 -> [w1069] mode=indexing
                      tunnel: [w1068] -> w1062 mode=indexing
                      i -> [w1070]
                      n769 = case shown="7" w1070 {
                        tunnel: [w1075 w1085 w1097 w1109 w1122] -> w1073
                        tunnel: w1072 -> [_ w1080 w1092 w1104 w1117]
                        tunnel: w1071 -> [w1075 w1082 w1094 w1106 w1119]
                        tunnel: w1069 -> [w1074 w1078 w1090 w1101 w1113]
                        tunnel: [w1074 FALSE ("布尔") FALSE ("布尔") FALSE ("布尔") FALSE ("布尔")] -> w1068
                        tunnel: 15 ("rank") -> [_ _ _ w1100 w1112]
                        tunnel: 2 ("rank") -> [_ w1077 w1089 _ _]
                        frame Default {
                        }
                        frame 4 {
                          n770 = global read "Global.vi" "工位一T1"() -> (w1079:dbl)
                          n771 = Unbundle(w1082) -> (w1084:dbl[], w1083:dbl[])
                          n772 = call <vilib>:"Median Filter PtByPt.vi"("initialize"=w1078) -> ()  [unwired: 3 in, 2 out]
                          n773 = Build Array (concatenate)(w1084, w1080) -> (w1087:dbl[])
                          n774 = call-poly <userlib>:"MGI Running Average.vi"("Averaging Size"=w1077, "Initialize? (F)"=w1078, "Value"=w1079) -> ("Average"=w1076:dbl)  [unwired: 8 in]
                          n775 = Build Array (concatenate)(w1083, w1076) -> (w1086:dbl[])
                          n776 = Bundle(w1087, w1086) -> (w1085:cluster{dbl[], dbl[]})  [unwired: 1 in]
                        }
                        frame 5 {
                          n777 = global read "Global.vi" "工位一T2"() -> (w1091:dbl)
                          n778 = Unbundle(w1094) -> (w1096:dbl[], w1095:dbl[])
                          n779 = call <vilib>:"Median Filter PtByPt.vi"("initialize"=w1090) -> ()  [unwired: 3 in, 2 out]
                          n780 = Build Array (concatenate)(w1096, w1092) -> (w1099:dbl[])
                          n781 = call-poly <userlib>:"MGI Running Average.vi"("Averaging Size"=w1089, "Initialize? (F)"=w1090, "Value"=w1091) -> ("Average"=w1088:dbl)  [unwired: 8 in]
                          n782 = Build Array (concatenate)(w1095, w1088) -> (w1098:dbl[])
                          n783 = Bundle(w1099, w1098) -> (w1097:cluster{dbl[], dbl[]})  [unwired: 1 in]
                        }
                        frame 6 {
                          n784 = call <vilib>:"Median Filter PtByPt.vi"("initialize"=w1101, "rank"=w1100, "x"=w1104) -> ()  [unwired: 1 in, 2 out]
                          n785 = Unbundle(w1106) -> (w1108:dbl[], w1107:dbl[])
                          n786 = global read "Global.vi" "工位一P"() -> (w1103:dbl)
                          n787 = Build Array (concatenate)(w1108, w1104) -> (w1111:dbl[])
                          n788 = call-poly <userlib>:"MGI Running Average.vi"("Averaging Size"=w1100, "Initialize? (F)"=w1101, "Value"=w1103) -> ("Average"=w1102:dbl)  [unwired: 8 in]
                          n789 = Build Array (concatenate)(w1107, w1102) -> (w1110:dbl[])
                          n790 = Bundle(w1111, w1110) -> (w1109:cluster{dbl[], dbl[]})  [unwired: 1 in]
                        }
                        frame 7 {
                          n791 = global read "Global.vi" "工位一S"() -> (w1115:dbl)
                          n792 = call <vilib>:"Median Filter PtByPt.vi"("initialize"=w1113, "rank"=w1112, "x"=w1117) -> ("Filtered x"=w1116:dbl)  [unwired: 1 in, 1 out]
                          n793 = Unbundle(w1119) -> (w1121:dbl[], w1120:dbl[])
                          n794 = Build Array (concatenate)(w1121, w1116) -> (w1124:dbl[])
                          n795 = call-poly <userlib>:"MGI Running Average.vi"("Averaging Size"=w1112, "Initialize? (F)"=w1113, "Value"=w1115) -> ("Average"=w1114:dbl)  [unwired: 8 in]
                          n796 = Build Array (concatenate)(w1120, w1114) -> (w1123:dbl[])
                          n797 = Bundle(w1124, w1123) -> (w1122:cluster{dbl[], dbl[]})  [unwired: 1 in]
                        }
                      }
                    }
                    n798 = local write "初始化 3"(w1062) -> ()
                    n799 = local write "动优化态前"(w1060) -> ()
                    n800 = call "VRES值.vi"("XY"=w1060, "索引1"=6, "索引2"=7) -> ("XY图 2"=w1061:cluster{dbl[], dbl[]}[])  [unwired: 16 in]
                    n801 = Index Array(array=w1061, index=8 ("索引")) -> (element=→"vRES_cCW":cluster{dbl[], dbl[]})
                  }
                  frame True {
                    n802 = call "传感器数据.vi"() -> ("传感器读数"=w1129:T6)  [unwired: 11 in]
                    n803 = Unbundle By Name(w1129) -> ("工位一驱动伺服位移"=w1125:sgl)
                    n804 = local read "可信度检测"() -> (w1130:cluster{dbl[], dbl[]}[])
                    n805 = local read "初始化 2"() -> (w1128:bool[])
                    n806 = for {
                      tunnel: [w1137] -> w1126 mode=indexing
                      tunnel: w1125 -> [w1136]
                      tunnel: w1130 -> [w1135] mode=indexing
                      tunnel: w1128 -> [w1133] mode=indexing
                      tunnel: [w1132] -> w1127 mode=indexing
                      i -> [w1134]
                      n807 = case shown="5" w1134 {
                        tunnel: [w1139 w1147 w1157 w1173] -> w1137
                        tunnel: w1136 -> [_ w1140 w1150 w1166]
                        tunnel: w1135 -> [w1139 w1144 w1154 w1170]
                        tunnel: w1133 -> [w1138 w1142 w1153 w1163]
                        tunnel: [w1138 FALSE ("布尔") FALSE ("布尔") FALSE ("布尔")] -> w1132
                        tunnel: 2 ("rank") -> [_ _ _ w1165]
                        frame Default {
                        }
                        frame 3 {
                          n808 = call <vilib>:"Median Filter PtByPt.vi"("initialize"=w1142) -> ()  [unwired: 3 in, 2 out]
                          n809 = Unbundle(w1144) -> (w1146:dbl[], w1145:dbl[])
                          n810 = global read "Global.vi" "工位一T1"() -> (w1141:dbl)
                          n811 = Build Array (concatenate)(w1146, w1140) -> (w1149:dbl[])
                          n812 = call <vilib>:"Median Filter PtByPt.vi"("initialize"=w1142) -> ()  [unwired: 3 in, 2 out]
                          n813 = Build Array (concatenate)(w1145, w1141) -> (w1148:dbl[])
                          n814 = Bundle(w1149, w1148) -> (w1147:cluster{dbl[], dbl[]})  [unwired: 1 in]
                        }
                        frame 4 {
                          n815 = Unbundle(w1154) -> (w1156:dbl[], w1155:dbl[])
                          n816 = call <vilib>:"Median Filter PtByPt.vi"("initialize"=w1153) -> ()  [unwired: 3 in, 2 out]
                          n817 = global read "Global.vi" "工位一T2"() -> (w1151:dbl)
                          n818 = Build Array (concatenate)(w1156, w1150) -> (w1159:dbl[])
                          n819 = call <vilib>:"Median Filter PtByPt.vi"("initialize"=w1153) -> ()  [unwired: 3 in, 2 out]
                          n820 = Build Array (concatenate)(w1155, w1151) -> (w1158:dbl[])
                          n821 = Bundle(w1159, w1158) -> (w1157:cluster{dbl[], dbl[]})  [unwired: 1 in]
                        }
                        frame 5 {
                          n822 = global read "Global.vi" "工位一P"() -> (w1167:dbl)
                          n823 = global read "Global.vi" "工位一S"() -> (w1168:dbl)
                          n824 = call <vilib>:"Median Filter PtByPt.vi"("initialize"=w1163, "rank"=w1165, "x"=w1166) -> ()  [unwired: 1 in, 2 out]
                          n825 = Unbundle(w1170) -> (w1172:dbl[], w1171:dbl[])
                          n826 = call "Calc_Vres.vi"("S_Data in"=w1168, "P_Data in"=w1167) -> ("Vres"=w1164:dbl)  [unwired: 7 in, 2 out]
                          n827 = Build Array (concatenate)(w1172, w1166) -> (w1175:dbl[])
                          n828 = call <vilib>:"Median Filter PtByPt.vi"("initialize"=w1163, "rank"=10, "x"=w1164) -> ("Filtered x"=w1161:dbl)  [unwired: 1 in, 1 out]
                          n829 = call-poly <userlib>:"MGI Running Average.vi"("Averaging Size"=w1165, "Initialize? (F)"=w1163, "Value"=w1161) -> ("Average"=w1162:dbl)  [unwired: 8 in]
                          n830 = Build Array (concatenate)(w1171, w1162) -> (w1174:dbl[])
                          n831 = Bundle(w1175, w1174) -> (w1173:cluster{dbl[], dbl[]})  [unwired: 1 in]
                        }
                      }
                    }
                    n832 = local write "可信度检测"(w1126) -> ()
                    n833 = local write "初始化 2"(w1127) -> ()
                  }
                }
                n834 = local read "initialize"() -> (w1054:bool)
                n835 = for {
                  N: 5 -> [_]
                  tunnel: w1054 -> [w1177]
                  tunnel: [w1178] -> w1053
                  i -> [w1176]
                  n836 = case shown="默认" w1176 {
                    tunnel: [w1179 FALSE ("initialize")] -> w1178
                    tunnel: w1177 -> [w1179 _]
                    frame Default {
                    }
                    frame 0 {
                    }
                  }
                }
                n837 = local write "initialize"(w1053) -> ()
              }
              frame 502 {
                n838 = global read "Global.vi" "动态优化完成"() -> (w1181:bool)
                n839 = case shown="真" w1181 {
                  frame False {
                    n840 = stacked-sequence {
                      frame #0 {
                        n841 = local read "动优化态前"() -> (w1182:cluster{dbl[], dbl[]}[])
                        n842 = for {
                          tunnel: w1182 -> [w1183] mode=indexing
                          i -> [w1184]
                          n843 = Unbundle(w1183) -> (w1185:dbl[])  [unwired: 1 out]
                          n844 = case shown="1" w1184 {
                            tunnel: w1185 -> [_ w1186 w1187 w1188 w1189 w1190 w1191 w1192 w1193]
                            frame Default {
                            }
                            frame 0 {
                              n845 = local write "T1_CW"(w1186) -> ()
                            }
                            frame 1 {
                              n846 = local write "T2_CW"(w1187) -> ()
                            }
                            frame 2 {
                              n847 = local write "P_CW"(w1188) -> ()
                            }
                            frame 3 {
                              n848 = local write "S_CW"(w1189) -> ()
                            }
                            frame 4 {
                              n849 = local write "T1_CCw"(w1190) -> ()
                            }
                            frame 5 {
                              n850 = local write "T2_CCw"(w1191) -> ()
                            }
                            frame 6 {
                              n851 = local write "P_CCw"(w1192) -> ()
                            }
                            frame 7 {
                              n852 = local write "S_CCw"(w1193) -> ()
                            }
                          }
                        }
                      }
                      frame #1 {
                        n853 = local read "T1_CCw"() -> (w1198:dbl[])
                        n854 = local read "T2_CCw"() -> (w1200:dbl[])
                        n855 = local read "T1_CW"() -> (w1196:dbl[])
                        n856 = local read "T2_CW"() -> (w1199:dbl[])
                        n857 = Build Array(w1199, w1200) -> (w1201:dbl[][])
                        n858 = local read "SENSOR"() -> (w1202:T1)
                        n859 = call-poly <userlib>:"MGI Average.vi"("Double[][]"=w1201, "Ignore NaN? (F)"=TRUE) -> ("Average"=w1204:dbl)
                        n860 = Build Array(w1196, w1198) -> (w1197:dbl[][])
                        n861 = local read "P_CCw"() -> (w1205:dbl[])
                        n862 = local read "S_CCw"() -> (w1207:dbl[])
                        n863 = local read "S_CW"() -> (w1208:dbl[])
                        n864 = local read "P_CW"() -> (w1206:dbl[])
                        n865 = call-poly <userlib>:"MGI Average.vi"("Double[][]"=w1197, "Ignore NaN? (F)"=TRUE) -> ("Average"=w1203:dbl)
                        n866 = call "动态优化.vi"("S_CCw"=w1207, "S_Cw"=w1208, "P_CCw"=w1205, "SENSOR"=w1202, "P_Cw"=w1206, "T2_AV(%)"=w1204, "T1_AV(%)"=w1203) -> ("OK？"=w1209:bool)  [unwired: 4 in]
                        n867 = case shown="真" w1209 {
                          selector: w1209 -> [_ w1217]
                          frame False {
                          }
                          frame True {
                            n868 = global read "Global.vi" "8点复测"() -> (w1213:bool)
                            n869 = global read "Global.vi" "动态优化复测"() -> (w1216:bool)
                            n870 = global write "Global.vi" "动态优化完成"(w1217) -> ()
                            n871 = Select(t="动态优化", s=w1216, f="复测") -> (s? t:f=w1212:string)
                            n872 = Select(t=w1212, s=w1213, f="复测判定") -> (s? t:f=w1210:string)
                            n873 = local write "STEP"(w1210) -> ()
                          }
                        }
                      }
                    }
                  }
                  frame True {
                    w1223 = FALSE ("工位二占空比采集")
                    n874 = local read "可信度检测"() -> (w1224:cluster{dbl[], dbl[]}[])
                    n875 = global write "Global.vi" "P/S采集"(w1223) -> ()
                    n876 = global write "Global.vi" "工位占空比采集"(w1223) -> ()
                    n877 = for {
                      tunnel: w1224 -> [w1225] mode=indexing
                      i -> [w1226]
                      n878 = Unbundle(w1225) -> (w1227:dbl[])  [unwired: 1 out]
                      n879 = case shown="2" w1226 {
                        tunnel: w1227 -> [_ w1228 w1229 _ w1231 w1232 _]
                        tunnel: w1225 -> [_ _ _ w1230 _ _ w1233]
                        frame Default {
                        }
                        frame 0 {
                          n880 = local write "T1_CW"(w1228) -> ()
                        }
                        frame 1 {
                          n881 = local write "T2_CW"(w1229) -> ()
                        }
                        frame 2 {
                          n882 = local write "VRES_cW"(w1230) -> ()
                        }
                        frame 3 {
                          n883 = local write "T1_CCw"(w1231) -> ()
                        }
                        frame 4 {
                          n884 = local write "T2_CCw"(w1232) -> ()
                        }
                        frame 5 {
                          n885 = local write "vRES_cCW"(w1233) -> ()
                        }
                      }
                    }
                    n886 = call "CloseVI.vi"("名称或相对路径"="PS采集优化.vi") -> ()  [unwired: 10 in, 1 out]
                    n887 = global read "Global.vi" "8点复测"() -> (w1222:bool)
                    n888 = Select(t="复测", s=w1222, f="复测判定") -> (s? t:f=w1220:string)
                    n889 = local write "STEP"(w1220) -> ()
                  }
                }
              }
              frame 505 {
                w1234 = TRUE ("initialize")
                n890 = local write "initialize"(w1234) -> ()
                n891 = local write "initialize 2"(w1234) -> ()
              }
              frame 511 {
                n892 = stacked-sequence {
                  frame #0 {
                    n893 = Wait (ms)(milliseconds to wait=u32 500 ("等待时间（毫秒）")) -> ()  [unwired: 1 out]
                  }
                  frame #1 {
                    w1245 = 10171 items=["上升"=10280, "下降"=10171] ("starting edge2")
                    w1244 = 10280 items=["上升"=10280, "下降"=10171] ("starting edge1")
                    w1246 = 10171 items=["上升"=10280, "下降"=10171] ("starting edge2")
                    w1247 = 10280 items=["上升"=10280, "下降"=10171] ("starting edge1")
                    w1254 = 10171 items=["上升"=10280, "下降"=10171] ("starting edge")
                    w1256 = 10171 items=["上升"=10280, "下降"=10171] ("starting edge")
                    w1255 = 10280 items=["上升"=10280, "下降"=10171] ("starting edge")
                    w1257 = 10280 items=["上升"=10280, "下降"=10171] ("starting edge")
                    n894 = local read "VRES_cW"() -> (w1253:cluster{dbl[], dbl[]})
                    n895 = Unbundle(w1253) -> (w1251:dbl[], w1250:dbl[])
                    n896 = call "占空比测量.vi"("计数器"=tag "Dev2/ctr6", "starting edge1"=w1257, "starting edge2"=w1256) -> ("占空比2(%)"=w1260:dbl)  [unwired: 4 in, 3 out]
                    n897 = call "占空比测量.vi"("计数器"=tag "Dev2/ctr7", "starting edge1"=w1255, "starting edge2"=w1254) -> ("占空比(%)"=w1259:dbl)  [unwired: 4 in, 3 out]
                    n898 = Threshold 1D Array(2:90.0 ("分数索引或x"), 3:w1251) -> (0:w1249:dbl)  [unwired: 1 in]
                    n899 = call "占空比测量.vi"("计数器"=tag "Dev2/ctr4", "starting edge1"=w1247, "starting edge2"=w1246) -> ("占空比2(%)"=w1242:dbl)  [unwired: 4 in, 3 out]
                    n900 = call "占空比测量.vi"("计数器"=tag "Dev2/ctr5", "starting edge1"=w1244, "starting edge2"=w1245) -> ("占空比2(%)"=w1241:dbl)  [unwired: 4 in, 3 out]
                    n901 = call "Calc_Vres.vi"("S_Data in"=w1259, "P_Data in"=w1260) -> ("Vres"=w1239:dbl)  [unwired: 7 in, 2 out]
                    n902 = Interpolate 1D Array(1:w1249, 2:w1250) -> (0:w1237:dbl)
                    n903 = Subtract(x=w1242, y=w1241) -> (x-y=→"T1-T2_90°":dbl)
                    n904 = Max & Min(x=w1237, y=w1239) -> (max(x,y)=w1238:dbl)  [unwired: 1 out]
                    n905 = local write "Vres_90°"(w1238) -> ()
                  }
                  frame #2 {
                    n906 = call "设备状态.vi"("枚举"=enum16{"Read", "Write"}."Write", "工位"=enum16{"工位一", "工位二"}."工位一", "Status_Write"=i16 512) -> ()  [unwired: 8 in, 1 out]
                  }
                }
                n907 = call "浮动通知.vi"("通知内容"="正向复测！" ("Status")) -> ()  [unwired: 11 in]
              }
              frame 513 {
                n908 = stacked-sequence {
                  frame #0 {
                    n909 = Wait (ms)(milliseconds to wait=u32 500 ("等待时间（毫秒）")) -> ()  [unwired: 1 out]
                  }
                  frame #1 {
                    w1274 = 10171 items=["上升"=10280, "下降"=10171] ("starting edge2")
                    w1273 = 10280 items=["上升"=10280, "下降"=10171] ("starting edge1")
                    w1275 = 10171 items=["上升"=10280, "下降"=10171] ("starting edge2")
                    w1276 = 10280 items=["上升"=10280, "下降"=10171] ("starting edge1")
                    w1283 = 10171 items=["上升"=10280, "下降"=10171] ("starting edge")
                    w1284 = 10280 items=["上升"=10280, "下降"=10171] ("starting edge")
                    w1285 = 10171 items=["上升"=10280, "下降"=10171] ("starting edge")
                    w1286 = 10280 items=["上升"=10280, "下降"=10171] ("starting edge")
                    n910 = local read "VRES_cW"() -> (w1282:cluster{dbl[], dbl[]})
                    n911 = Unbundle(w1282) -> (w1280:dbl[], w1279:dbl[])
                    n912 = call "占空比测量.vi"("计数器"=tag "Dev2/ctr6", "starting edge1"=w1286, "starting edge2"=w1285) -> ("占空比2(%)"=w1288:dbl)  [unwired: 4 in, 3 out]
                    n913 = call "占空比测量.vi"("计数器"=tag "Dev2/ctr7", "starting edge1"=w1284, "starting edge2"=w1283) -> ("占空比(%)"=w1287:dbl)  [unwired: 4 in, 3 out]
                    n914 = Threshold 1D Array(2:180.0 ("分数索引或x"), 3:w1280) -> (0:w1278:dbl)  [unwired: 1 in]
                    n915 = call "Calc_Vres.vi"("S_Data in"=w1287, "P_Data in"=w1288) -> ("Vres"=w1267:dbl)  [unwired: 7 in, 2 out]
                    n916 = Interpolate 1D Array(1:w1278, 2:w1279) -> (0:w1266:dbl)
                    n917 = call "占空比测量.vi"("计数器"=tag "Dev2/ctr4", "starting edge1"=w1276, "starting edge2"=w1275) -> ("占空比2(%)"=w1271:dbl)  [unwired: 4 in, 3 out]
                    n918 = call "占空比测量.vi"("计数器"=tag "Dev2/ctr5", "starting edge1"=w1273, "starting edge2"=w1274) -> ("占空比2(%)"=w1270:dbl)  [unwired: 4 in, 3 out]
                    n919 = Subtract(x=w1271, y=w1270) -> (x-y=→"T1-T2_180°":dbl)
                    n920 = Max & Min(x=w1266, y=w1267) -> (max(x,y)=w1268:dbl)  [unwired: 1 out]
                    n921 = local write "Vres_180°"(w1268) -> ()
                  }
                  frame #2 {
                    n922 = call "设备状态.vi"("枚举"=enum16{"Read", "Write"}."Write", "工位"=enum16{"工位一", "工位二"}."工位一", "Status_Write"=i16 514) -> ()  [unwired: 8 in, 1 out]
                  }
                }
              }
              frame 515 {
                n923 = stacked-sequence {
                  frame #0 {
                    n924 = Wait (ms)(milliseconds to wait=u32 500 ("等待时间（毫秒）")) -> ()  [unwired: 1 out]
                  }
                  frame #1 {
                    w1303 = 10171 items=["上升"=10280, "下降"=10171] ("starting edge2")
                    w1302 = 10280 items=["上升"=10280, "下降"=10171] ("starting edge1")
                    w1304 = 10171 items=["上升"=10280, "下降"=10171] ("starting edge2")
                    w1305 = 10280 items=["上升"=10280, "下降"=10171] ("starting edge1")
                    w1312 = 10171 items=["上升"=10280, "下降"=10171] ("starting edge")
                    w1313 = 10280 items=["上升"=10280, "下降"=10171] ("starting edge")
                    w1314 = 10171 items=["上升"=10280, "下降"=10171] ("starting edge")
                    w1315 = 10280 items=["上升"=10280, "下降"=10171] ("starting edge")
                    n925 = local read "VRES_cW"() -> (w1311:cluster{dbl[], dbl[]})
                    n926 = Unbundle(w1311) -> (w1309:dbl[], w1308:dbl[])
                    n927 = call "占空比测量.vi"("计数器"=tag "Dev2/ctr6", "starting edge1"=w1315, "starting edge2"=w1314) -> ("占空比2(%)"=w1317:dbl)  [unwired: 4 in, 3 out]
                    n928 = call "占空比测量.vi"("计数器"=tag "Dev2/ctr7", "starting edge1"=w1313, "starting edge2"=w1312) -> ("占空比(%)"=w1316:dbl)  [unwired: 4 in, 3 out]
                    n929 = Threshold 1D Array(2:270.0 ("分数索引或x"), 3:w1309) -> (0:w1307:dbl)  [unwired: 1 in]
                    n930 = call "Calc_Vres.vi"("S_Data in"=w1316, "P_Data in"=w1317) -> ("Vres"=w1295:dbl)  [unwired: 7 in, 2 out]
                    n931 = call "占空比测量.vi"("计数器"=tag "Dev2/ctr4", "starting edge1"=w1305, "starting edge2"=w1304) -> ("占空比2(%)"=w1300:dbl)  [unwired: 4 in, 3 out]
                    n932 = call "占空比测量.vi"("计数器"=tag "Dev2/ctr5", "starting edge1"=w1302, "starting edge2"=w1303) -> ("占空比2(%)"=w1299:dbl)  [unwired: 4 in, 3 out]
                    n933 = Interpolate 1D Array(1:w1307, 2:w1308) -> (0:w1296:dbl)
                    n934 = Subtract(x=w1300, y=w1299) -> (x-y=→"T1-T2_270°":dbl)
                    n935 = Max & Min(x=w1296, y=w1295) -> (max(x,y)=w1297:dbl)  [unwired: 1 out]
                    n936 = local write "Vres_270°"(w1297) -> ()
                  }
                  frame #2 {
                    n937 = call "设备状态.vi"("枚举"=enum16{"Read", "Write"}."Write", "工位"=enum16{"工位一", "工位二"}."工位一", "Status_Write"=i16 516) -> ()  [unwired: 8 in, 1 out]
                  }
                }
              }
              frame 517 {
                n938 = stacked-sequence {
                  frame #0 {
                    n939 = Wait (ms)(milliseconds to wait=u32 500 ("等待时间（毫秒）")) -> ()  [unwired: 1 out]
                  }
                  frame #1 {
                    w1332 = 10171 items=["上升"=10280, "下降"=10171] ("starting edge2")
                    w1331 = 10280 items=["上升"=10280, "下降"=10171] ("starting edge1")
                    w1333 = 10171 items=["上升"=10280, "下降"=10171] ("starting edge2")
                    w1334 = 10280 items=["上升"=10280, "下降"=10171] ("starting edge1")
                    w1341 = 10171 items=["上升"=10280, "下降"=10171] ("starting edge")
                    w1342 = 10280 items=["上升"=10280, "下降"=10171] ("starting edge")
                    w1343 = 10171 items=["上升"=10280, "下降"=10171] ("starting edge")
                    w1344 = 10280 items=["上升"=10280, "下降"=10171] ("starting edge")
                    n940 = local read "VRES_cW"() -> (w1340:cluster{dbl[], dbl[]})
                    n941 = Unbundle(w1340) -> (w1338:dbl[], w1337:dbl[])
                    n942 = call "占空比测量.vi"("计数器"=tag "Dev2/ctr6", "starting edge1"=w1344, "starting edge2"=w1343) -> ("占空比2(%)"=w1346:dbl)  [unwired: 4 in, 3 out]
                    n943 = call "占空比测量.vi"("计数器"=tag "Dev2/ctr7", "starting edge1"=w1342, "starting edge2"=w1341) -> ("占空比(%)"=w1345:dbl)  [unwired: 4 in, 3 out]
                    n944 = Threshold 1D Array(2:360.0 ("分数索引或x"), 3:w1338) -> (0:w1336:dbl)  [unwired: 1 in]
                    n945 = call "Calc_Vres.vi"("S_Data in"=w1345, "P_Data in"=w1346) -> ("Vres"=w1324:dbl)  [unwired: 7 in, 2 out]
                    n946 = call "占空比测量.vi"("计数器"=tag "Dev2/ctr4", "starting edge1"=w1334, "starting edge2"=w1333) -> ("占空比2(%)"=w1329:dbl)  [unwired: 4 in, 3 out]
                    n947 = call "占空比测量.vi"("计数器"=tag "Dev2/ctr5", "starting edge1"=w1331, "starting edge2"=w1332) -> ("占空比2(%)"=w1328:dbl)  [unwired: 4 in, 3 out]
                    n948 = Interpolate 1D Array(1:w1336, 2:w1337) -> (0:w1325:dbl)
                    n949 = Subtract(x=w1329, y=w1328) -> (x-y=→"T1-T2_360°":dbl)
                    n950 = Max & Min(x=w1325, y=w1324) -> (max(x,y)=w1326:dbl)  [unwired: 1 out]
                    n951 = local write "Vres_360°"(w1326) -> ()
                  }
                  frame #2 {
                    n952 = call "设备状态.vi"("枚举"=enum16{"Read", "Write"}."Write", "工位"=enum16{"工位一", "工位二"}."工位一", "Status_Write"=i16 520) -> ()  [unwired: 8 in, 1 out]
                  }
                }
              }
              frame 521 {
                n953 = stacked-sequence {
                  frame #0 {
                    n954 = Wait (ms)(milliseconds to wait=u32 500 ("等待时间（毫秒）")) -> ()  [unwired: 1 out]
                  }
                  frame #1 {
                    w1362 = 10171 items=["上升"=10280, "下降"=10171] ("starting edge2")
                    w1361 = 10280 items=["上升"=10280, "下降"=10171] ("starting edge1")
                    w1363 = 10171 items=["上升"=10280, "下降"=10171] ("starting edge2")
                    w1364 = 10280 items=["上升"=10280, "下降"=10171] ("starting edge1")
                    w1373 = 10171 items=["上升"=10280, "下降"=10171] ("starting edge")
                    w1374 = 10280 items=["上升"=10280, "下降"=10171] ("starting edge")
                    w1375 = 10171 items=["上升"=10280, "下降"=10171] ("starting edge")
                    w1376 = 10280 items=["上升"=10280, "下降"=10171] ("starting edge")
                    n955 = local read "vRES_cCW"() -> (w1372:cluster{dbl[], dbl[]})
                    n956 = Unbundle(w1372) -> (w1369:dbl[], w1367:dbl[])
                    n957 = call "占空比测量.vi"("计数器"=tag "Dev2/ctr6", "starting edge1"=w1376, "starting edge2"=w1375) -> ("占空比2(%)"=w1378:dbl)  [unwired: 4 in, 3 out]
                    n958 = call "占空比测量.vi"("计数器"=tag "Dev2/ctr7", "starting edge1"=w1374, "starting edge2"=w1373) -> ("占空比(%)"=w1377:dbl)  [unwired: 4 in, 3 out]
                    n959 = Reverse 1D Array(array=w1369) -> (reversed array=w1368:dbl[])
                    n960 = Threshold 1D Array(2:315.0 ("分数索引或x"), 3:w1368) -> (0:w1370:dbl)  [unwired: 1 in]
                    n961 = call "Calc_Vres.vi"("S_Data in"=w1377, "P_Data in"=w1378) -> ("Vres"=w1354:dbl)  [unwired: 7 in, 2 out]
                    n962 = Reverse 1D Array(array=w1367) -> (reversed array=w1366:dbl[])
                    n963 = call "占空比测量.vi"("计数器"=tag "Dev2/ctr4", "starting edge1"=w1364, "starting edge2"=w1363) -> ("占空比2(%)"=w1359:dbl)  [unwired: 4 in, 3 out]
                    n964 = call "占空比测量.vi"("计数器"=tag "Dev2/ctr5", "starting edge1"=w1361, "starting edge2"=w1362) -> ("占空比2(%)"=w1358:dbl)  [unwired: 4 in, 3 out]
                    n965 = Interpolate 1D Array(1:w1370, 2:w1366) -> (0:w1355:dbl)
                    n966 = Subtract(x=w1359, y=w1358) -> (x-y=→"T1-T2_315°":dbl)
                    n967 = Max & Min(x=w1354, y=w1355) -> (max(x,y)=w1356:dbl)  [unwired: 1 out]
                    n968 = local write "Vres_315°"(w1356) -> ()
                  }
                  frame #2 {
                    n969 = call "设备状态.vi"("枚举"=enum16{"Read", "Write"}."Write", "工位"=enum16{"工位一", "工位二"}."工位一", "Status_Write"=i16 522) -> ()  [unwired: 8 in, 1 out]
                  }
                }
                n970 = call "浮动通知.vi"("通知内容"="逆向复测！" ("Status")) -> ()  [unwired: 11 in]
              }
              frame 523 {
                n971 = stacked-sequence {
                  frame #0 {
                    n972 = Wait (ms)(milliseconds to wait=u32 500 ("等待时间（毫秒）")) -> ()  [unwired: 1 out]
                  }
                  frame #1 {
                    w1393 = 10171 items=["上升"=10280, "下降"=10171] ("starting edge2")
                    w1392 = 10280 items=["上升"=10280, "下降"=10171] ("starting edge1")
                    w1394 = 10171 items=["上升"=10280, "下降"=10171] ("starting edge2")
                    w1395 = 10280 items=["上升"=10280, "下降"=10171] ("starting edge1")
                    w1404 = 10171 items=["上升"=10280, "下降"=10171] ("starting edge")
                    w1405 = 10280 items=["上升"=10280, "下降"=10171] ("starting edge")
                    w1406 = 10171 items=["上升"=10280, "下降"=10171] ("starting edge")
                    w1407 = 10280 items=["上升"=10280, "下降"=10171] ("starting edge")
                    n973 = local read "vRES_cCW"() -> (w1403:cluster{dbl[], dbl[]})
                    n974 = Unbundle(w1403) -> (w1400:dbl[], w1398:dbl[])
                    n975 = Reverse 1D Array(array=w1400) -> (reversed array=w1399:dbl[])
                    n976 = call "占空比测量.vi"("计数器"=tag "Dev2/ctr6", "starting edge1"=w1407, "starting edge2"=w1406) -> ("占空比2(%)"=w1409:dbl)  [unwired: 4 in, 3 out]
                    n977 = call "占空比测量.vi"("计数器"=tag "Dev2/ctr7", "starting edge1"=w1405, "starting edge2"=w1404) -> ("占空比(%)"=w1408:dbl)  [unwired: 4 in, 3 out]
                    n978 = Threshold 1D Array(2:225.0 ("分数索引或x"), 3:w1399) -> (0:w1401:dbl)  [unwired: 1 in]
                    n979 = Reverse 1D Array(array=w1398) -> (reversed array=w1397:dbl[])
                    n980 = call "Calc_Vres.vi"("S_Data in"=w1408, "P_Data in"=w1409) -> ("Vres"=w1385:dbl)  [unwired: 7 in, 2 out]
                    n981 = Interpolate 1D Array(1:w1401, 2:w1397) -> (0:w1386:dbl)
                    n982 = call "占空比测量.vi"("计数器"=tag "Dev2/ctr4", "starting edge1"=w1395, "starting edge2"=w1394) -> ("占空比2(%)"=w1390:dbl)  [unwired: 4 in, 3 out]
                    n983 = call "占空比测量.vi"("计数器"=tag "Dev2/ctr5", "starting edge1"=w1392, "starting edge2"=w1393) -> ("占空比2(%)"=w1389:dbl)  [unwired: 4 in, 3 out]
                    n984 = Subtract(x=w1390, y=w1389) -> (x-y=→"T1-T2_225°":dbl)
                    n985 = Max & Min(x=w1386, y=w1385) -> (max(x,y)=w1387:dbl)  [unwired: 1 out]
                    n986 = local write "Vres_225°"(w1387) -> ()
                  }
                  frame #2 {
                    n987 = call "设备状态.vi"("枚举"=enum16{"Read", "Write"}."Write", "工位"=enum16{"工位一", "工位二"}."工位一", "Status_Write"=i16 524) -> ()  [unwired: 8 in, 1 out]
                  }
                }
              }
              frame 525 {
                n988 = stacked-sequence {
                  frame #0 {
                    n989 = Wait (ms)(milliseconds to wait=u32 500 ("等待时间（毫秒）")) -> ()  [unwired: 1 out]
                  }
                  frame #1 {
                    w1424 = 10171 items=["上升"=10280, "下降"=10171] ("starting edge2")
                    w1423 = 10280 items=["上升"=10280, "下降"=10171] ("starting edge1")
                    w1425 = 10171 items=["上升"=10280, "下降"=10171] ("starting edge2")
                    w1426 = 10280 items=["上升"=10280, "下降"=10171] ("starting edge1")
                    w1435 = 10171 items=["上升"=10280, "下降"=10171] ("starting edge")
                    w1436 = 10280 items=["上升"=10280, "下降"=10171] ("starting edge")
                    w1437 = 10171 items=["上升"=10280, "下降"=10171] ("starting edge")
                    w1438 = 10280 items=["上升"=10280, "下降"=10171] ("starting edge")
                    n990 = local read "vRES_cCW"() -> (w1434:cluster{dbl[], dbl[]})
                    n991 = Unbundle(w1434) -> (w1429:dbl[], w1431:dbl[])
                    n992 = Reverse 1D Array(array=w1429) -> (reversed array=w1428:dbl[])
                    n993 = call "占空比测量.vi"("计数器"=tag "Dev2/ctr6", "starting edge1"=w1438, "starting edge2"=w1437) -> ("占空比2(%)"=w1440:dbl)  [unwired: 4 in, 3 out]
                    n994 = call "占空比测量.vi"("计数器"=tag "Dev2/ctr7", "starting edge1"=w1436, "starting edge2"=w1435) -> ("占空比(%)"=w1439:dbl)  [unwired: 4 in, 3 out]
                    n995 = Threshold 1D Array(2:135.0 ("分数索引或x"), 3:w1428) -> (0:w1432:dbl)  [unwired: 1 in]
                    n996 = Reverse 1D Array(array=w1431) -> (reversed array=w1430:dbl[])
                    n997 = call "Calc_Vres.vi"("S_Data in"=w1439, "P_Data in"=w1440) -> ("Vres"=w1417:dbl)  [unwired: 7 in, 2 out]
                    n998 = Interpolate 1D Array(1:w1432, 2:w1430) -> (0:w1416:dbl)
                    n999 = call "占空比测量.vi"("计数器"=tag "Dev2/ctr4", "starting edge1"=w1426, "starting edge2"=w1425) -> ("占空比2(%)"=w1421:dbl)  [unwired: 4 in, 3 out]
                    n1000 = call "占空比测量.vi"("计数器"=tag "Dev2/ctr5", "starting edge1"=w1423, "starting edge2"=w1424) -> ("占空比2(%)"=w1420:dbl)  [unwired: 4 in, 3 out]
                    n1001 = Max & Min(x=w1416, y=w1417) -> (max(x,y)=w1418:dbl)  [unwired: 1 out]
                    n1002 = Subtract(x=w1421, y=w1420) -> (x-y=→"T1-T2_135°":dbl)
                    n1003 = local write "Vres_135°"(w1418) -> ()
                  }
                  frame #2 {
                    n1004 = call "设备状态.vi"("枚举"=enum16{"Read", "Write"}."Write", "工位"=enum16{"工位一", "工位二"}."工位一", "Status_Write"=i16 526) -> ()  [unwired: 8 in, 1 out]
                  }
                }
              }
              frame 527 {
                n1005 = stacked-sequence {
                  frame #0 {
                    n1006 = Wait (ms)(milliseconds to wait=u32 500 ("等待时间（毫秒）")) -> ()  [unwired: 1 out]
                  }
                  frame #1 {
                    w1453 = 10171 items=["上升"=10280, "下降"=10171] ("starting edge2")
                    w1454 = 10280 items=["上升"=10280, "下降"=10171] ("starting edge1")
                    w1450 = 10171 items=["上升"=10280, "下降"=10171] ("starting edge2")
                    w1451 = 10280 items=["上升"=10280, "下降"=10171] ("starting edge1")
                    w1466 = 10171 items=["上升"=10280, "下降"=10171] ("starting edge")
                    w1467 = 10280 items=["上升"=10280, "下降"=10171] ("starting edge")
                    w1468 = 10171 items=["上升"=10280, "下降"=10171] ("starting edge")
                    w1469 = 10280 items=["上升"=10280, "下降"=10171] ("starting edge")
                    n1007 = local read "vRES_cCW"() -> (w1465:cluster{dbl[], dbl[]})
                    n1008 = Unbundle(w1465) -> (w1461:dbl[], w1460:dbl[])
                    n1009 = call "占空比测量.vi"("计数器"=tag "Dev2/ctr6", "starting edge1"=w1469, "starting edge2"=w1468) -> ("占空比2(%)"=w1471:dbl)  [unwired: 4 in, 3 out]
                    n1010 = call "占空比测量.vi"("计数器"=tag "Dev2/ctr7", "starting edge1"=w1467, "starting edge2"=w1466) -> ("占空比(%)"=w1470:dbl)  [unwired: 4 in, 3 out]
                    n1011 = Reverse 1D Array(array=w1461) -> (reversed array=w1462:dbl[])
                    n1012 = call "Calc_Vres.vi"("S_Data in"=w1470, "P_Data in"=w1471) -> ("Vres"=w1448:dbl)  [unwired: 7 in, 2 out]
                    n1013 = Reverse 1D Array(array=w1460) -> (reversed array=w1459:dbl[])
                    n1014 = Threshold 1D Array(2:45.0 ("分数索引或x"), 3:w1462) -> (0:w1464:dbl)  [unwired: 1 in]
                    n1015 = Interpolate 1D Array(1:w1464, 2:w1459) -> (0:w1447:dbl)
                    n1016 = Max & Min(x=w1447, y=w1448) -> (max(x,y)=w1449:dbl)  [unwired: 1 out]
                    n1017 = call "占空比测量.vi"("计数器"=tag "Dev2/ctr4", "starting edge1"=w1451, "starting edge2"=w1450) -> ("占空比2(%)"=w1458:dbl)  [unwired: 4 in, 3 out]
                    n1018 = call "占空比测量.vi"("计数器"=tag "Dev2/ctr5", "starting edge1"=w1454, "starting edge2"=w1453) -> ("占空比2(%)"=w1457:dbl)  [unwired: 4 in, 3 out]
                    n1019 = local write "Vres_45°"(w1449) -> ()
                    n1020 = Subtract(x=w1458, y=w1457) -> (x-y=→"T1-T2_45°":dbl)
                  }
                  frame #2 {
                    n1021 = local write "STEP"("复测判定") -> ()
                  }
                }
              }
              frame 530 {
              }
              frame 1024 {
                n1022 = local write "STEP"("退出自动" ("STEP")) -> ()
              }
            }
          }
          frame "不合格" {
            n1023 = local write "STEP"("等待" ("STEP")) -> ()
            n1024 = Wait (ms)(milliseconds to wait=u32 100 ("等待时间（毫秒）")) -> ()  [unwired: 1 out]
            n1025 = call "设备状态.vi"("枚举"=enum16{"Read", "Write"}."Write", "工位"=enum16{"工位一", "工位二"}."工位一", "Status_Write"=i16 400) -> ()  [unwired: 8 in, 1 out]
          }
          frame "报表" {
            n1026 = stacked-sequence {
              frame #0 {
                n1027 = global write "Global.vi" "计时开始"(FALSE ("计时开始")) -> ()
              }
              frame #1 {
                n1028 = disable-structure shown="禁用" {
                  frame Disabled {
                    n1029 = global read "Global.vi" "产品编号"() -> (w1490:string)
                    n1030 = Concatenate Strings("graph\\" ("名称或相对路径"), w1490, ".hsg" ("字符串")) -> (w1491:string)
                    n1031 = call <vilib>:"Application Directory.vi"() -> ("Application Directory"=w1493:path)
                    n1032 = local read "动优化态前"() -> (w1497:cluster{dbl[], dbl[]}[])
                    n1033 = local read "传感器特性"() -> (w1482:cluster{dbl[], dbl[]}[])
                    n1034 = local read "可信度检测"() -> (w1498:cluster{dbl[], dbl[]}[])
                    n1035 = Build Path(base path=w1493, name or relative path=w1491) -> (appended path=w1486:path)
                    n1036 = Bundle("可信度检测"=w1498, "动优化态前"=w1497, "传感器特性"=w1482) -> (w1496:T10)  [unwired: 1 in]
                    n1037 = Open/Create/Replace File(file path (use dialog)=w1486, operation (0:open)=T5."open or create" ("操作(0:open)")) -> (refnum out=w1484:refnum<file>, error out=w1483:errorcluster)  [unwired: 4 in, 1 out]
                    n1038 = Flatten To JSON(anything=w1496, error in (no error)=w1483) -> (JSON string=w1495:string, 11:w1494:errorcluster)  [unwired: 1 in]
                    n1039 = Write to Binary File(file (use dialog)=w1484, data=w1495, error in=w1494) -> (refnum out=w1487:refnum<file>, error out=w1488:errorcluster)  [unwired: 3 in, 1 out]
                    n1040 = Close File(refnum=w1487, error in=w1488) -> ()  [unwired: 2 out]
                  }
                  frame Enabled {
                  }
                }
              }
              frame #2 {
                n1041 = global read "Global.vi" "工位"() -> (w1504:enum16{"左工位", "右工位"})
                n1042 = call "时间秒.vi"() -> ("结果字符串"=w1502:string)  [unwired: 11 in]
                n1043 = global read "Global.vi" "产品编号"() -> (w1501:string)
                n1044 = call <vilib>:"Space Constant.vi"() -> ("String"=w1499:string)
                n1045 = case shown="\"左工位\", 默认" w1504 {
                  tunnel: ["左工位" ("工位名称") _] -> w1503
                  frame "左工位", Default {
                  }
                  frame "右工位" {
                  }
                }
                n1046 = Concatenate Strings(w1501, w1499, w1502) -> (w1500:string)
                n1047 = call "Report.vi"("文件重命名"=TRUE, "文件名称"=w1500, "工位名称"=w1503, "判定结果"="判定结果") -> ("RESULT_VALUE"=w1505:string)  [unwired: 6 in, 1 out]
                n1048 = global read "Global.vi" "联机模式"() -> (w1508:enum16{"单机", "追溯"})
                n1049 = case shown="\"追溯\"" w1508 {
                  tunnel: w1505 -> [_ w1510]
                  frame "单机", Default {
                  }
                  frame "追溯" {
                    n1050 = global read "Global.vi" "Result"() -> (w1515:refnum<vi>)
                    n1051 = property class="Tbl"(reference=w1515) -> (reference out=w1514:refnum<vi>, "Row Headers[]"=w1512:string[])  [unwired: 1 in, 1 out]
                    n1052 = property class="Tbl"(reference=w1514) -> ("Value"=w1513:string[][])  [unwired: 1 in, 2 out]
                    n1053 = for {
                      tunnel: w1513 -> [w1521] mode=indexing
                      tunnel: w1512 -> [w1522] mode=indexing
                      tunnel: [w1519] -> w1511 mode=indexing if=w1520
                      n1054 = Index Array(array=w1521) -> (element=w1523:string)  [unwired: 1 in]
                      n1055 = Build Array (concatenate)(w1522, w1521) -> (w1519:string[])
                      n1056 = case shown="\"\"" w1523 {
                        tunnel: [TRUE FALSE] -> w1520
                        frame Default {
                        }
                        frame "" {
                        }
                      }
                    }
                    n1057 = global read "追溯Global.vi" "DEVICE_ID"() -> (w1517:string)
                    n1058 = global read "追溯Global.vi" "CODE_ID"() -> (w1516:string)
                    n1059 = global read "追溯Global.vi" "USER_ID"() -> (w1518:string)
                    n1060 = call "UPRESULT.vi"("DEVICE_ID"=w1517, "USER_ID"=w1518, "CODE_ID"=w1516, "RESULT_VALUE"=w1510) -> ()  [unwired: 11 in, 1 out]
                    n1061 = call "UPTEST.vi"("Result"=w1511, "CODE_ID"=w1516, "DEVICE_ID"=w1517) -> ()  [unwired: 6 in, 1 out]
                  }
                }
              }
              frame #3 {
                n1062 = local write "STEP"("进入自动" ("STEP")) -> ()
              }
            }
          }
        }
        n1063 = global read "Global.vi" "程序关闭"() -> (w15:bool)
      }
      n1064 = while {
        stop <- w1527 stop-if-true
        n1065 = event shown="[4] \"传感器特性\": 鼠标进入;  \"传感器特性\": 鼠标离开;  \"传感器特性\": 游标移动" {
          selector: _ -> [_ _ _ _ _ _]
          dyn-events: _ -> [_ _ _ _ _ _]
          timeout: 1000 -> [_ _ _ _ _ _]
          event Timeout {
            n1066 = event-data() -> ()  [unwired: 1 in, 3 out]
            n1067 = call "Obtain Broadcast Events for Registration.vi"() -> ("Already running?"=w1529:bool)  [unwired: 9 in, 2 out]
            n1068 = case shown="真" w1529 {
              frame False {
                n1069 = local write "STEP"("手动" ("STEP")) -> ()
              }
              frame True {
                n1070 = call "错误代码.vi"() -> ("Status_Read"=w1531:u32)  [unwired: 11 in]
                n1071 = feedback #9() -> (w1541:u32)  [unwired: 1 in]
                n1072 = feedback-in #9(w1531) -> ()
                n1073 = case shown="0" w1531 {
                  frame 0 {
                    n1074 = global read "Global.vi" "报警图标"() -> (w1542:refnum<vi>)
                    n1075 = property class="Bool"(reference=w1542, "Visible"=FALSE ("可见")) -> ()  [unwired: 1 in, 2 out]
                  }
                  frame 1, Default {
                    n1076 = global read "Global.vi" "报警图标"() -> (w1545:refnum<vi>)
                    n1077 = property class="Bool"(reference=w1545, "Visible"=TRUE ("可见")) -> ()  [unwired: 1 in, 2 out]
                  }
                }
                n1078 = Greater Or Equal?(x=w1531, y=i16 5000) -> (x >= y?=w1539:bool)
                n1079 = Less?(x=w1531, y=i16 5200) -> (x < y?=w1540:bool)
                n1080 = Equal?(x=w1531, y=w1541) -> (x = y?=w1538:bool)
                n1081 = global read "Global.vi" "报警图标"() -> (w1533:refnum<vi>)
                n1082 = And(x=w1539, y=w1540) -> (x .and. y?=w1532:bool)
                n1083 = property class="Bool"(reference=w1533, "Value"=w1532) -> ()  [unwired: 1 in, 2 out]
                n1084 = Bundle By Name(cluster=errorcluster {"status"=FALSE, "code"=0, "source"=""} ("错误常量"), "status"=w1532, "code"=w1531) -> (w1537:errorcluster)
                n1085 = case shown="假" w1538 {
                  tunnel: w1537 -> [w1546 _]
                  frame False {
                    n1086 = call "报警处理.vi"("错误常量"=w1546) -> ()  [unwired: 9 in, 2 out]
                  }
                  frame True {
                  }
                }
              }
            }
          }
          event Menu Selection (User) {
            n1087 = event-data() -> ("ItemTag"=w1547:string)  [unwired: 1 in, 2 out]
            n1088 = case shown="\"真\"" w1547 {
              frame "假", Default {
              }
              frame "真" {
              }
            }
          }
          event "传感器特性": Scale Range Change {
            n1089 = event-data() -> ("CtlRef"=w1548:refnum<vi>)  [unwired: 1 in]
            n1090 = call "XY_conf备份.vi"("方式"=enum16{"写入", "读取"}."写入", "XY图引用"=w1548) -> ()  [unwired: 3 in, 1 out]
          }
          event Panel Close {
            n1091 = event-data() -> ()  [unwired: 1 in, 4 out]
            n1092 = global write "Global.vi" "程序关闭"(TRUE ("程序关闭")) -> ()
          }
          event "传感器特性": Mouse Enter; "传感器特性": Mouse Leave; "传感器特性": Cursor Move {
            n1093 = event-data() -> ("CtlRef"=w1553:refnum<vi>, "Type"=w1551:T11)  [unwired: 1 in]
            n1094 = call "CursorShow.vi"("nameShow"=TRUE, "Type"=w1551, "Graph"=w1553) -> ()  [unwired: 7 in, 2 out]
          }
          event "传感器特性", "可信度检测": Mouse Down {
            n1095 = event-data() -> ("CtlRef"=w1558:refnum<vi>, "Coords"=w1557:T12, "Type"=w1555:T11)  [unwired: 1 in]
            n1096 = invoke class="XYGraph (严格)" method="Map Coords To XY"(reference=w1558, "Coords"=w1557) -> (reference out=w1556:refnum<vi>, "XY"=w1554:cluster{"X":dbl, "Y":dbl})  [unwired: 5 in, 5 out]
            n1097 = call "CursorShow.vi"("游标.游标位置"=w1554, "Type"=w1555, "Graph"=w1556) -> ()  [unwired: 7 in, 2 out]
          }
        }
        n1098 = global read "Global.vi" "程序关闭"() -> (w1527:bool)
      }
    }
  }
